vi "Live Capture Functional Stack.11.64bit.vi"() -> ()   [LabVIEW 2014]
uses:
  subvis/Stack Track.ctl
  subvis/Stack_State.ctl
  CameraControlTypeDef.ctl
  Desktop/camtiff/ctiff.llb/__CTIFFNewFileAndStyleUINT16.vi
  Desktop/camtiff/ctiff.llb/__CTIFFAddNewPageUINT16.vi
panel:
  out "Video":T1(plugin-control)
  out "Internal Line Interval":dbl
  in  "Mode":bool
  in  "Preview":bool
  in  "Capture Mode":bool
  out "Record Ready":bool
  in  "Stacks":dbl=1.0
  out "Stack Frames":i32=100
  in  "Stack Frames":i32=100
  in  "Temp":path=path "C:/temp.tmp"
  in  "Frames":i32=100
  in  "HardDisk Record":bool
  in  "Internal Line Interval":dbl
  in  "Slit Width / Lines":sgl=150.0
  in  "Camera Readout Mode":u16(ring)=12 items=["Full Frame"=1, "Slit Scanning"=12]
  in  "Readout Direction":sgl(ring)=1.0 items=["Forward"=1, "Backward"=2]
  in  "Trigger Mode":sgl(ring)=1.0 items=["Normal"=1, "Start "=6]
  in  "Trigger Source":sgl(ring)=2.0 items=["Internal"=1, "External"=2]
  out "State":T2=enum."Start Sequence"
  out "Saving":bool
  in  "AutoIncrement":bool=TRUE
  in  "Path":path=path "C:/Users/spim/Desktop/Craig Cap/temp/a.tiff"
  in  "Frames":i32=100
  out "Frame Index":i32
  out "error out":errorcluster
  in  "stop":bool
  in  "Ram Record":bool
  out "Total Frames":i32
  out "Elapsed Time":u32
  out "Software FPS":dbl
  out "Camera FPS":dbl
  in  "H Offset":i32 min=0 max=0 step=4
  in  "H Width":i32 min=4 max=2048 step=4
  out "SMD":dbl
  out "SHO":i32
  in  "V Offset":i32 min=0 max=0 step=4
  in  "V Width":i32 min=4 max=2048 step=4
  in  "Binning":u16(ring) items=["1x1"=1, "2x2"=2, "4x4"=4]
  out "SHW":i32
  out "SVO":i32
  out "SVW":i32
  in  "Scan Mode":dbl min=1.0 max=2.0 step=1.0
  in  "Exposure":dbl min=0.0010036691729323308 max=10.000004210526315 step=1e-08
  out "EXP":dbl
  out "Camera Model":string
  out "Camera Version":string
  out "Camera Serial":string
  # "Capture Mode"
  # "Preview Mode"
  # "HDD superior, will not drop frames or stacks"
  # "Change to rock switch"
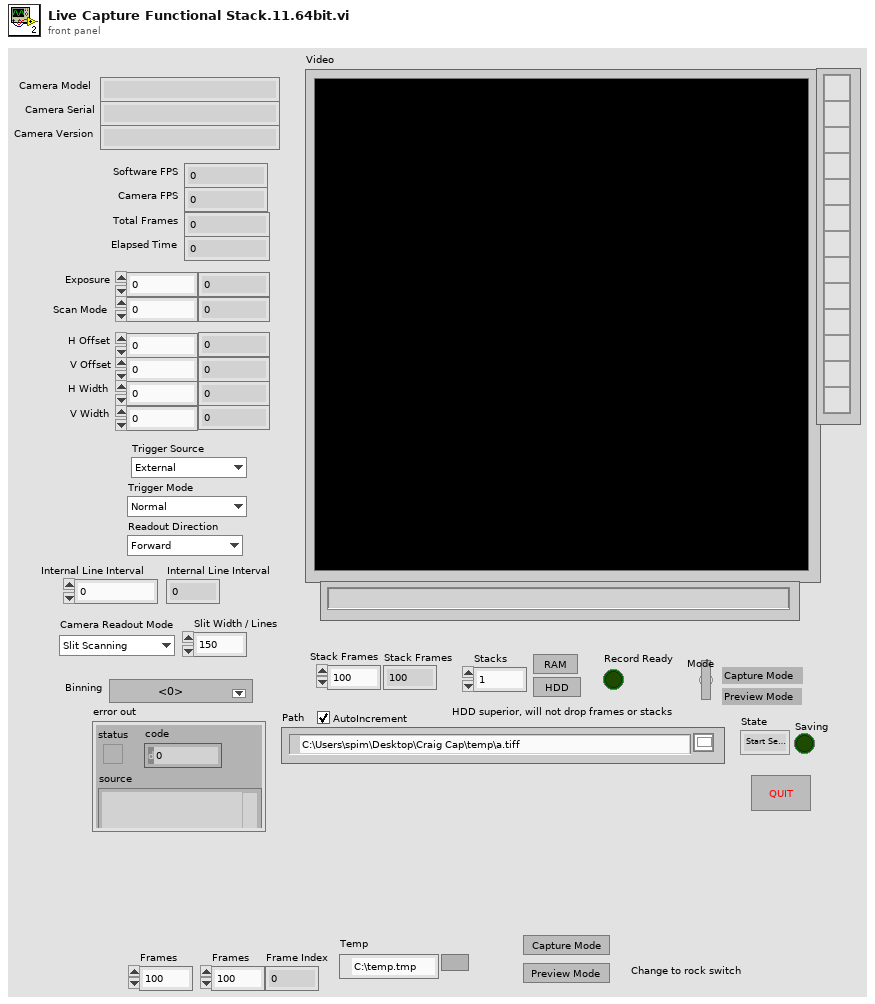
[diagram p1: front panel]
types:
  T1 = typedef "IMAQ Image.ctl" = refnum<image>
  T2 = typedef "Stack Track.ctl" = enum16{"Idle", "Start Sequence", "Read Disk", "STOP", "Collecting", "End"}
  T3 = typedef "CameraControlTypeDef.ctl" = enum16{"IntervalLineInt", "Ram Record", "HardDisk Record", "Disengage Update", "Update", "Idle", "ROI", "Binning", "Scan Mode", "Trigger Mode", "Readout Mode", "Readout Direction", "Preview"}
  T4 = typedef "Stack_State.ctl" = cluster{"State":T2, "Stack Number":i32, "Image":u16[][], "Stacks":i32}
  T5 = enum8{"Enabled", "Disabled", "Disabled and Grayed Out"}
  T6 = typedef "Image Type" = u32
  T7 = cluster{"Model":string, "Camera ID":string, "Firmware":string}
  T8 = cluster{"Value":i32, "Minimum":i32, "Maximum":i32, "Increment":i32}
  T9 = cluster{"height":u32, "width":u32, "datatype":u32}
  T10 = cluster{"H Offset":i32, "V Offset":i32, "H Width":i32, "V Width":i32}
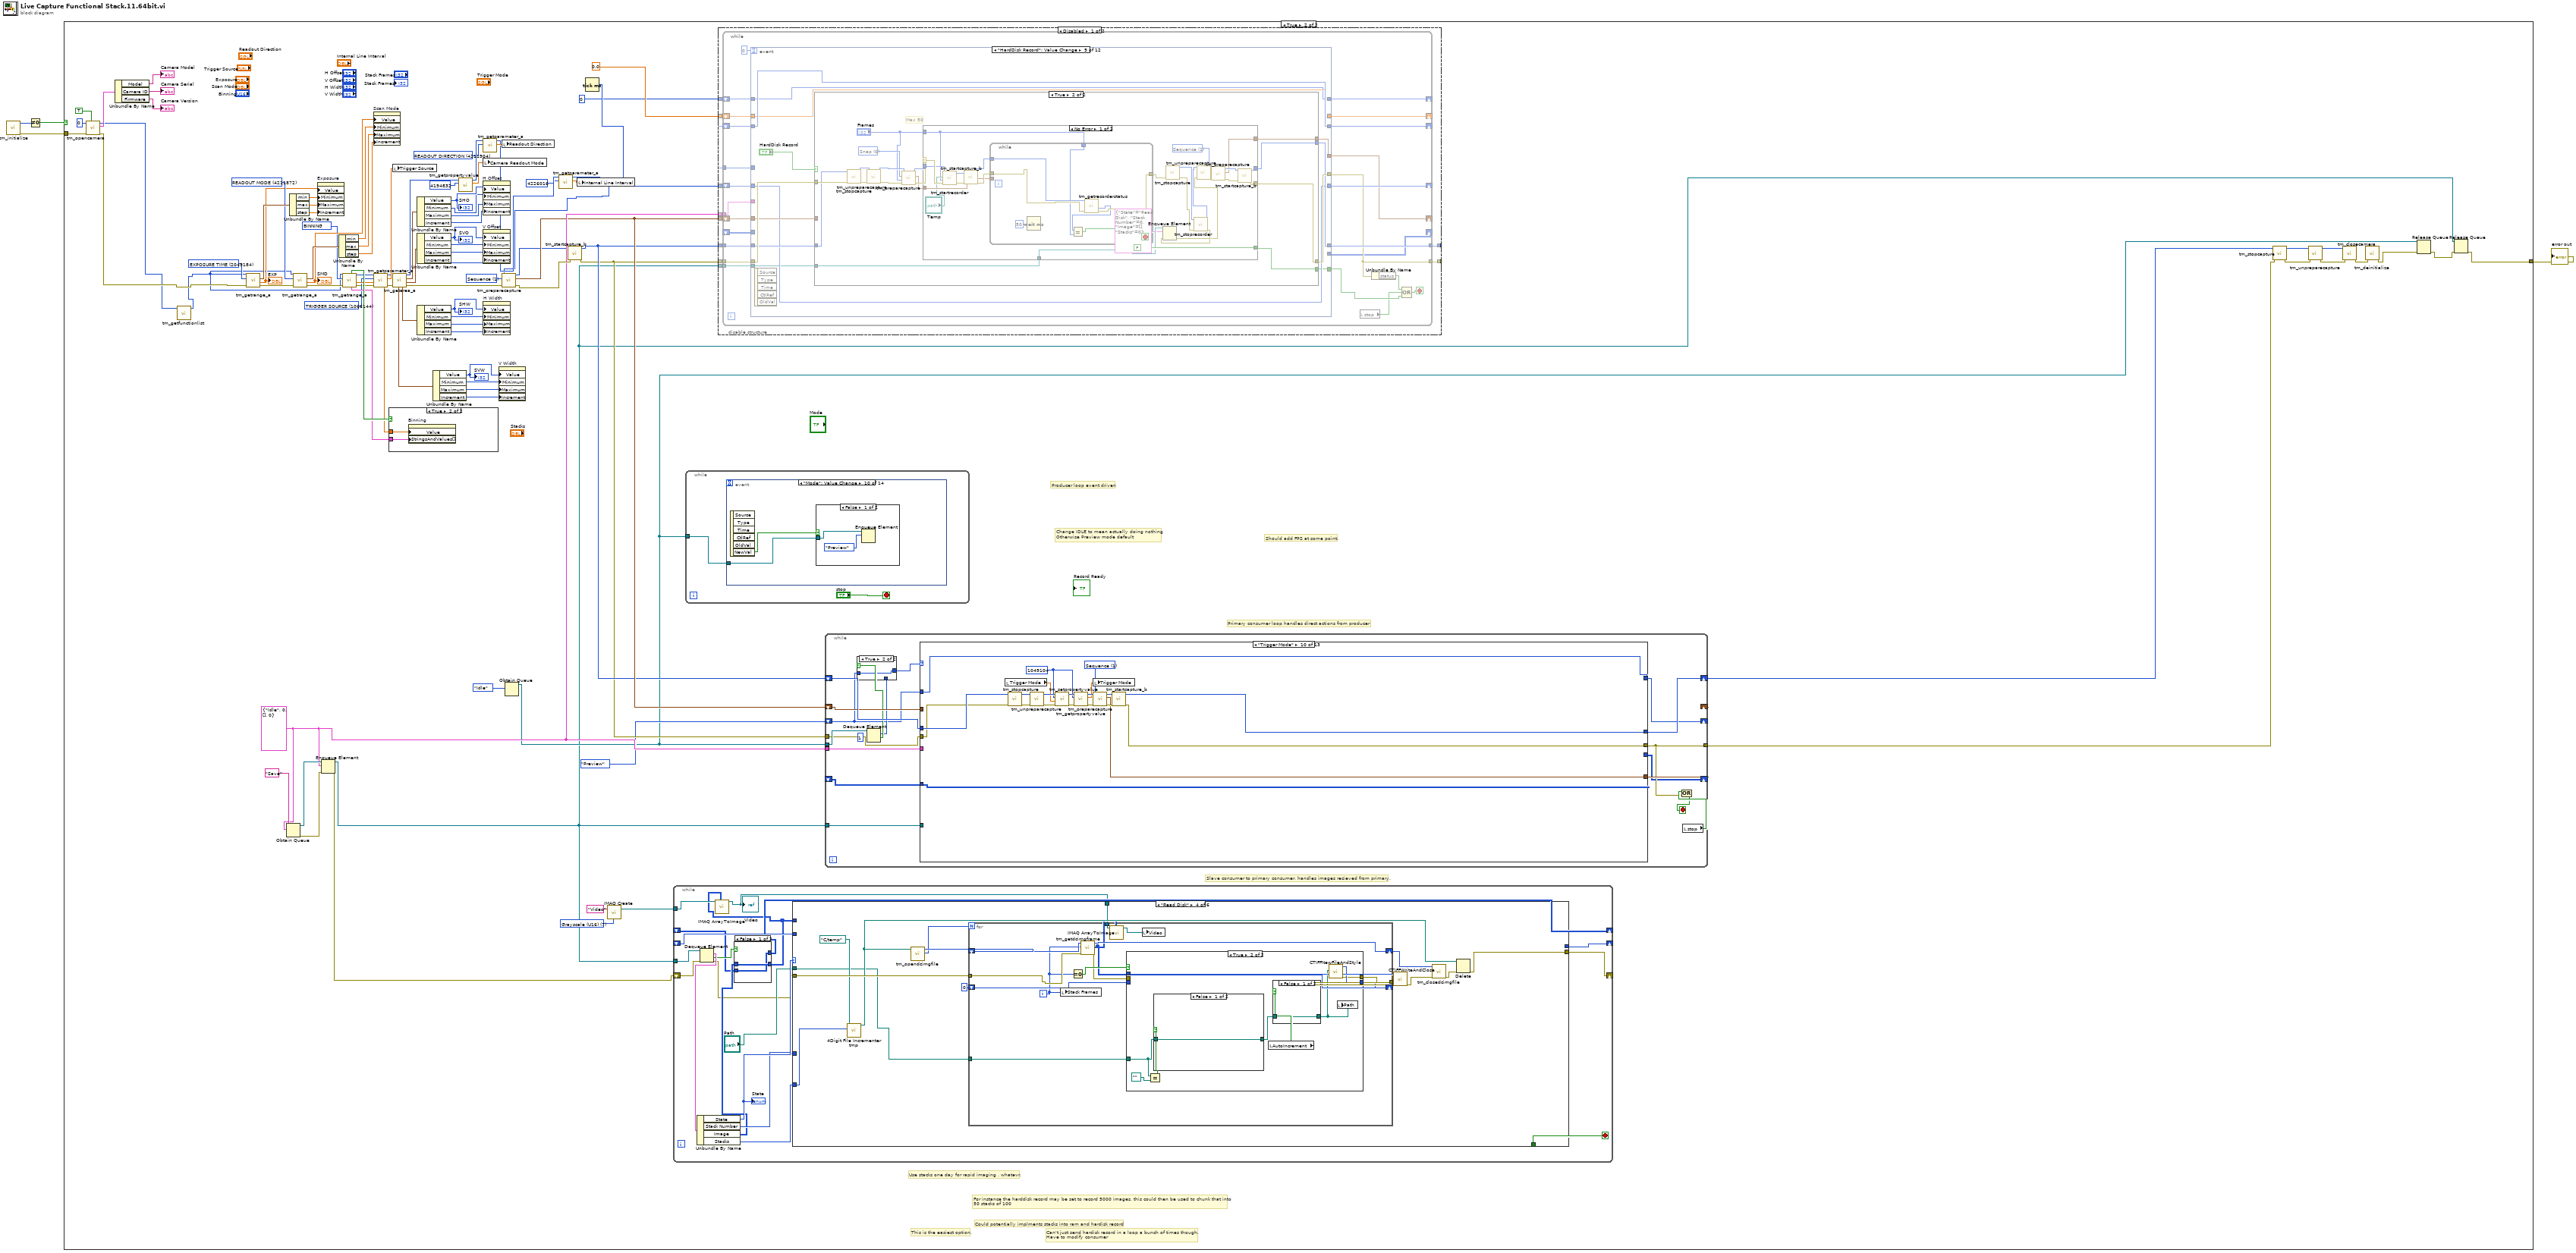
[diagram p0: block diagram]
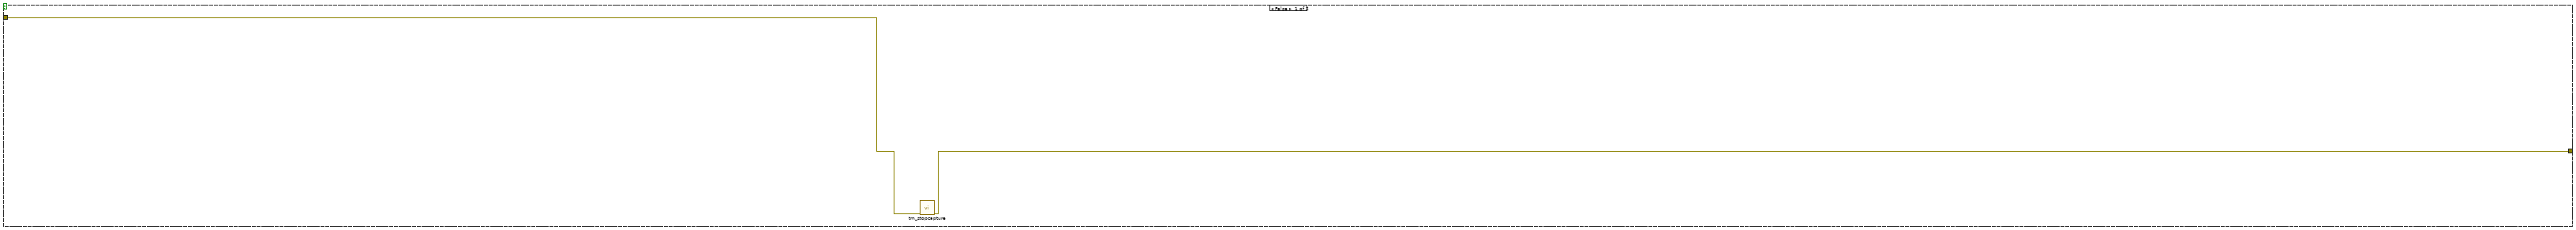
[diagram p2: hidden frame]
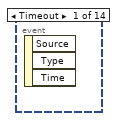
[diagram p3: hidden frame]
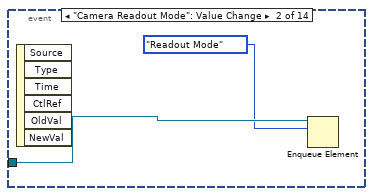
[diagram p4: hidden frame]
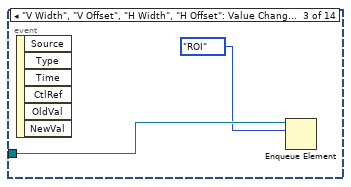
[diagram p5: hidden frame]
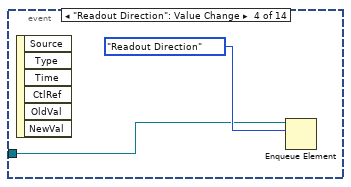
[diagram p6: hidden frame]
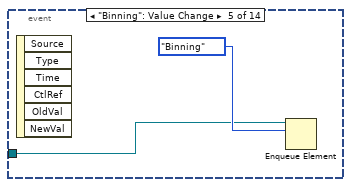
[diagram p7: hidden frame]
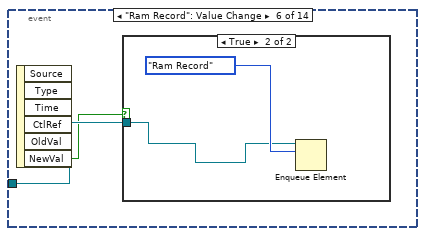
[diagram p8: hidden frame]
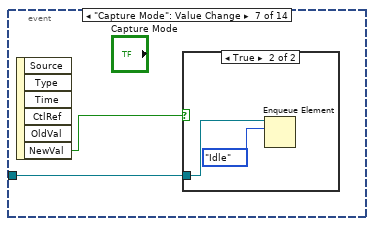
[diagram p10: hidden frame]
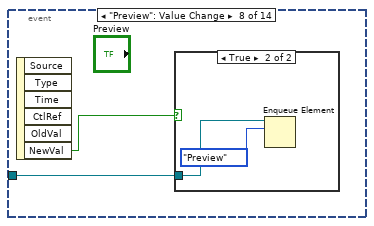
[diagram p12: hidden frame]
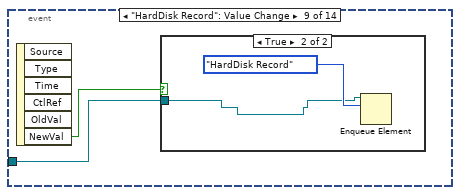
[diagram p14: hidden frame]
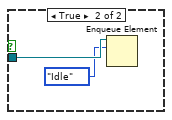
[diagram p16: hidden frame]
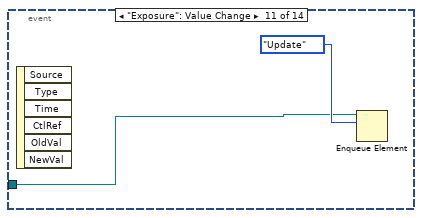
[diagram p17: hidden frame]
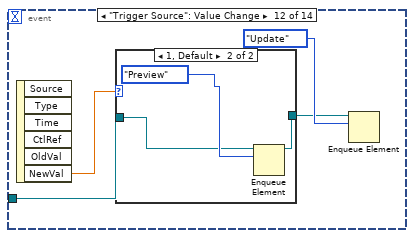
[diagram p18: hidden frame]
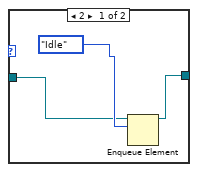
[diagram p19: hidden frame]
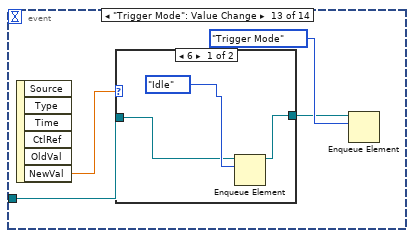
[diagram p20: hidden frame]
diagram:
  n1 = call <userlib>:"tm_initialize.vi"() -> ("error out"=w2:errorcluster, "Number Of Cameras"=w1:u32)  [unwired: 8 in, 2 out]
  n2 = Not Equal To 0?(x=w1) -> (x != 0?=w4:bool)
  n3 = case shown="True" w4 {
    tunnel: [w5 w19] -> w3
    tunnel: w2 -> [w6 w102]
    frame False {
      n4 = call <userlib>:"tm_stopcapture.vi"("error in (no error)"=w6) -> ("error out"=w5:errorcluster)  [unwired: 9 in, 1 out]
    }
    frame True {
      w9 = T6 7 items=["Grayscale (U8)", "Grayscale (I16)", "Grayscale (SGL)", "Complex (CSG)", "RGB (U32)", "HSL (U32)", "RGB (U64)", "Grayscale (U16)"] ("Image Type")
      w37 = u32 4211904 items=["SENSOR MODE"=4212128, "CCD MODE"=4212384, "READOUT MODE"=4211872, "ACTIVE VIEW INDEX"=4343136, "BITS PER CHANNEL"=4342976, "IMAGE PIXEL TYPE"=4343296, "BINNING"=4215968, "EXPOSURE TIME"=2049184, "CONTRAST GAIN"=3163312, "CONTRAST OFFSET"=3163328, "LIGHT MODE"=2114720, "SENSITIVITY"=2114992, "PHOTON IMAGING MODE"=2115200, "HIGH DYNAMIC RANGE MODE"=3163360, "WHITE BALANCE"=3163568, "TEMPERATURE"=2115232, "TEMPERATURE TARGET"=2115264, "SENSOR COOLER FAN"=2115296, "LINEBUNDLE HEIGHT"=4212192, "MECHANICAL SHUTTER"=2115488, "BACK FOCUS POSITION"=8422304, "TRIGGER CONNECTOR"=1066432, "TRIGGER SOURCE"=1066144, "OUTPUT TRIGGER SOURCE"=1852576, "TRIGGER GLOBAL EXPOSURE"=2049680, "FIRST TRIGGER BEHAVIOR"=2049696, "CHANNEL SYNC"=1852352, "READOUT DIRECTION"=4211904, "PRE HSYNC COUNT"=1852704] ("Parameter")
      w46 = u32 1066144 items=["SENSOR MODE"=4212128, "CCD MODE"=4212384, "READOUT MODE"=4211872, "ACTIVE VIEW INDEX"=4343136, "BITS PER CHANNEL"=4342976, "IMAGE PIXEL TYPE"=4343296, "BINNING"=4215968, "EXPOSURE TIME"=2049184, "CONTRAST GAIN"=3163312, "CONTRAST OFFSET"=3163328, "LIGHT MODE"=2114720, "SENSITIVITY"=2114992, "PHOTON IMAGING MODE"=2115200, "HIGH DYNAMIC RANGE MODE"=3163360, "WHITE BALANCE"=3163568, "TEMPERATURE"=2115232, "TEMPERATURE TARGET"=2115264, "SENSOR COOLER FAN"=2115296, "LINEBUNDLE HEIGHT"=4212192, "MECHANICAL SHUTTER"=2115488, "BACK FOCUS POSITION"=8422304, "TRIGGER CONNECTOR"=1066432, "TRIGGER SOURCE"=1066144, "OUTPUT TRIGGER SOURCE"=1852576, "TRIGGER GLOBAL EXPOSURE"=2049680, "FIRST TRIGGER BEHAVIOR"=2049696, "CHANNEL SYNC"=1852352, "READOUT DIRECTION"=4211904, "PRE HSYNC COUNT"=1852704] ("Parameter")
      w32 = T4 {"State"=enum."Idle", "Stack Number"=0, "Image"=[], "Stacks"=0} ("input cluster")
      w51 = u32 2049184 items=["BINNING"=4215968, "BITS PER CHANNEL"=4342976, "ACTIVE VIEW INDEX"=4343136, "CCD MODE"=4212384, "SENSOR MODE"=4212128, "READOUT MODE"=4211872, "EXPOSURE TIME"=2049184, "CONTRAST GAIN"=3163312, "CONTRAST OFFSET"=3163328, "LIGHT MODE"=2114720, "SENSITIVITY"=2114992, "WHITE BALANCE"=3163568, "PHOTON IMAGING MODE"=2115200, "HIGH DYNAMIC RANGE MODE"=3163360, "TRIGGER SOURCE"=1066144, "TRIGGER ACTIVE"=1066160, "TRIGGER MODE"=1066400, "TRIGGER POLARITY"=1066416, "TRIGGER GLOBAL EXPOSURE"=2049680, "FIRST TRIGGER BEHAVIOR"=2049696, "TRIGGER TIMES"=1066448, "OUTPUT TRIGGER POLARITY"=1852592, "OUTPUT TRIGGER DELAY"=1852624, "OUTPUT TRIGGER PERIOD"=1852640, "TEMPERATURE"=2115232, "TEMPERATURE TARGET"=2115264, "SENSOR COOLER FAN"=2115296, "MECHANICAL SHUTTER"=2115488, "BACK FOCUS POSITION"=8422304, "FRAMEBUNDLE MODE"=4346784, "FRAMEBUNDLE NUMBER"=4346800, "LINEBUNDLE HEIGHT"=4212192, "TRIGGER CONNECTOR"=1066432, "IMAGE PIXEL TYPE"=4343296, "OUTPUT TRIGGER KIND"=1852656, "READOUT DIRECTION"=4211904, "CHANNEL SYNC"=1852352] ("Parameter")
      w52 = u32 4211872 items=["BINNING"=4215968, "BITS PER CHANNEL"=4342976, "ACTIVE VIEW INDEX"=4343136, "CCD MODE"=4212384, "SENSOR MODE"=4212128, "READOUT MODE"=4211872, "EXPOSURE TIME"=2049184, "CONTRAST GAIN"=3163312, "CONTRAST OFFSET"=3163328, "LIGHT MODE"=2114720, "SENSITIVITY"=2114992, "WHITE BALANCE"=3163568, "PHOTON IMAGING MODE"=2115200, "HIGH DYNAMIC RANGE MODE"=3163360, "TRIGGER SOURCE"=1066144, "TRIGGER ACTIVE"=1066160, "TRIGGER MODE"=1066400, "TRIGGER POLARITY"=1066416, "TRIGGER GLOBAL EXPOSURE"=2049680, "FIRST TRIGGER BEHAVIOR"=2049696, "TRIGGER TIMES"=1066448, "OUTPUT TRIGGER POLARITY"=1852592, "OUTPUT TRIGGER DELAY"=1852624, "OUTPUT TRIGGER PERIOD"=1852640, "TEMPERATURE"=2115232, "TEMPERATURE TARGET"=2115264, "SENSOR COOLER FAN"=2115296, "MECHANICAL SHUTTER"=2115488, "BACK FOCUS POSITION"=8422304, "FRAMEBUNDLE MODE"=4346784, "FRAMEBUNDLE NUMBER"=4346800, "LINEBUNDLE HEIGHT"=4212192, "TRIGGER CONNECTOR"=1066432, "IMAGE PIXEL TYPE"=4343296, "OUTPUT TRIGGER KIND"=1852656, "READOUT DIRECTION"=4211904, "CHANNEL SYNC"=1852352] ("Parameter")
      w53 = u32 4215968 items=["BINNING"=4215968, "BITS PER CHANNEL"=4342976, "ACTIVE VIEW INDEX"=4343136, "CCD MODE"=4212384, "SENSOR MODE"=4212128, "READOUT MODE"=4211872, "EXPOSURE TIME"=2049184, "CONTRAST GAIN"=3163312, "CONTRAST OFFSET"=3163328, "LIGHT MODE"=2114720, "SENSITIVITY"=2114992, "WHITE BALANCE"=3163568, "PHOTON IMAGING MODE"=2115200, "HIGH DYNAMIC RANGE MODE"=3163360, "TRIGGER SOURCE"=1066144, "TRIGGER ACTIVE"=1066160, "TRIGGER MODE"=1066400, "TRIGGER POLARITY"=1066416, "TRIGGER GLOBAL EXPOSURE"=2049680, "FIRST TRIGGER BEHAVIOR"=2049696, "TRIGGER TIMES"=1066448, "OUTPUT TRIGGER POLARITY"=1852592, "OUTPUT TRIGGER DELAY"=1852624, "OUTPUT TRIGGER PERIOD"=1852640, "TEMPERATURE"=2115232, "TEMPERATURE TARGET"=2115264, "SENSOR COOLER FAN"=2115296, "MECHANICAL SHUTTER"=2115488, "BACK FOCUS POSITION"=8422304, "FRAMEBUNDLE MODE"=4346784, "FRAMEBUNDLE NUMBER"=4346800, "LINEBUNDLE HEIGHT"=4212192, "TRIGGER CONNECTOR"=1066432, "IMAGE PIXEL TYPE"=4343296, "OUTPUT TRIGGER KIND"=1852656, "READOUT DIRECTION"=4211904, "CHANNEL SYNC"=1852352] ("Parameter")
      w98 = 1 items=["Snap", "Sequence"] ("Capture mode")
      # "Can't just send hardisk record in a loop a bunch of times though.\nHave to modify consumer"
      # "This is the easiest option."
      # "Could potentially implments stacks into ram and hardisk record"
      # "For instance the harddisk record may be set to record 5000 images, this could then be used to chunk that into\n50 stacks of 100"
      # "Use stacks one day for rapid imaging , whatevr."
      # "Change IDLE to mean actually doing nothing\nOtherwise Preview mode default"
      # "Slave consumer to primary consumer, handles images recieved from primary."
      # "Primary consumer loop handles direct actions from producer"
      # "Producer loop event driven"
      # "Should add FPS at some point."
      n5 = call <userlib>:"tm_opencamera.vi"("Force Open"=TRUE, "error in (no error)"=w102, "Camera Index"=u32 0) -> ("error out"=w33:errorcluster, "Camera Details"=w65:T7, "Handle out"=w17:u32)  [unwired: 6 in]
      n6 = Unbundle By Name(w65) -> ("Model"=→"Camera Model":string, "Camera ID"=→"Camera Serial":string, "Firmware"=→"Camera Version":string)
      n7 = call <userlib>:"tm_getfunctionlist.vi"("Handle in"=w17) -> ("Handle out"=w16:u32)  [unwired: 8 in, 2 out]
      n8 = call <userlib>:"tm_getrange_a.vi"("error in (no error)"=w33, "Parameter"=w51, "Handle in"=w16) -> ("error out"=w60:errorcluster, "default"=w49:dbl, "Range"=w61:cluster{"min":dbl, "max":dbl, "step":dbl})  [unwired: 2 in, 4 out]
      "EXP" <- w49
      n9 = Obtain Queue(name (unnamed)="Save", element data type=w32) -> (queue out=w35:refnum<queue>, error out=w14:errorcluster)  [unwired: 3 in, 1 out]
      n10 = Unbundle By Name(w61) -> ("min"=w96:dbl, "max"=w95:dbl, "step"=w94:dbl)
      n11 = call <userlib>:"tm_getrange_a.vi"("error in (no error)"=w60, "Parameter"=w52, "Handle in"=w16) -> ("error out"=w57:errorcluster, "default"=w58:dbl, "Range"=w59:cluster{"min":dbl, "max":dbl, "step":dbl})  [unwired: 2 in, 4 out]
      "SMD" <- w58
      n12 = property on="Exposure" class="DigNum (strict)"("Value"=w49, "Minimum"=w96, "Maximum"=w95, "Increment"=w94) -> ()  [unwired: 2 in, 2 out]
      n13 = Enqueue Element(queue=w35, element=w32, error in (no error)=w14) -> (queue out=w18:refnum<queue>, error out=w13:errorcluster)  [unwired: 1 in, 1 out]
      n14 = Unbundle By Name(w59) -> ("min"=w93:dbl, "max"=w92:dbl, "step"=w91:dbl)
      n15 = call <userlib>:"tm_getrange_a.vi"("error in (no error)"=w57, "Parameter"=w53, "Handle in"=w16) -> ("error out"=w43:errorcluster, "default"=w55:dbl, "Handle out"=w45:u32, "Value Names"=w54:cluster{"Name":string, "Value":dbl}[], "Writable"=w56:bool)  [unwired: 2 in, 2 out]
      n16 = property on="Scan Mode" class="DigNum (strict)"("Value"=w58, "Minimum"=w93, "Maximum"=w92, "Increment"=w91) -> ()  [unwired: 2 in, 2 out]
      n17 = call <userlib>:"tm_getparameter_a.vi"("error in (no error)"=w43, "Parameter"=w46, "Handle in"=w45) -> ("error out"=w42:errorcluster, "Value out"=w47:dbl, "Handle out"=w44:u32)  [unwired: 6 in]
      n18 = case shown="True" w56 {
        tunnel: w54 -> [_ w1206]
        tunnel: w55 -> [_ w1205]
        frame False {
        }
        frame True {
          n19 = property on="Binning" class="Ring (strict)"("Value"=w1205, "StringsAndValues[]"=w1206) -> ()  [unwired: 2 in, 2 out]
        }
      }
      n20 = local write "Trigger Source"(w47) -> ()
      n21 = call <userlib>:"tm_getarea_a.vi"("error in (no error)"=w42, "Handle in"=w44) -> ("error out"=w48:errorcluster, "V Offset"=w90:T8, "H Offset"=w71:T8, "Handle out"=w39:u32, "H Width"=w89:T8, "V Width"=w88:T8)  [unwired: 4 in]
      n22 = Unbundle By Name(w71) -> ("Value"=w70:i32, "Minimum"=w69:i32, "Maximum"=w68:i32, "Increment"=w67:i32)
      "SHO" <- w70
      n23 = Unbundle By Name(w90) -> ("Value"=w78:i32, "Minimum"=w87:i32, "Maximum"=w86:i32, "Increment"=w85:i32)
      "SVO" <- w78
      n24 = Unbundle By Name(w89) -> ("Value"=w77:i32, "Minimum"=w84:i32, "Maximum"=w83:i32, "Increment"=w82:i32)
      "SHW" <- w77
      n25 = Unbundle By Name(w88) -> ("Value"=w76:i32, "Minimum"=w81:i32, "Maximum"=w80:i32, "Increment"=w79:i32)
      "SVW" <- w76
      n26 = call <userlib>:"tm_getpropertyvalue.vi"("Property ID"=u32 4194832, "Handle in"=w39) -> ("Value in"=w40:sgl, "Handle out"=w38:u32)  [unwired: 7 in, 1 out]
      n27 = call <userlib>:"tm_getparameter_a.vi"("Parameter"=w37, "Handle in"=w38) -> ("Value out"=w36:dbl, "Handle out"=w23:u32)  [unwired: 7 in, 1 out]
      n28 = local write "Camera Readout Mode"(w40) -> ()
      n29 = property on="H Offset" class="DigNum (strict)"("Value"=w70, "Minimum"=w69, "Maximum"=w68, "Increment"=w67) -> ()  [unwired: 2 in, 2 out]
      n30 = property on="V Offset" class="DigNum (strict)"("Value"=w78, "Minimum"=w87, "Maximum"=w86, "Increment"=w85) -> ()  [unwired: 2 in, 2 out]
      n31 = property on="H Width" class="DigNum (strict)"("Value"=w77, "Minimum"=w84, "Maximum"=w83, "Increment"=w82) -> ()  [unwired: 2 in, 2 out]
      n32 = property on="V Width" class="DigNum (strict)"("Value"=w76, "Minimum"=w81, "Maximum"=w80, "Increment"=w79) -> ()  [unwired: 2 in, 2 out]
      n33 = local write "Readout Direction"(w36) -> ()
      n34 = Obtain Queue(element data type=CameraControlTypeDef."Idle" ("Enum")) -> (queue out=w21:refnum<queue>)  [unwired: 4 in, 2 out]
      n35 = call <userlib>:"tm_getparameter_a.vi"("Parameter"=4226016, "Handle in"=w23) -> ("Value out"=w11:dbl, "Handle out"=w12:u32)  [unwired: 7 in, 1 out]
      n36 = call <userlib>:"tm_preparecapture.vi"("error in (no error)"=w48, "Capture mode"=w98, "Handle in"=w12) -> ("error out"=w34:errorcluster, "Buffer Info"=w31:T9, "Handle out"=w24:u32)  [unwired: 5 in, 1 out]
      n37 = call <userlib>:"tm_startcapture_b.vi"("error in (no error)"=w34, "Handle in"=w24) -> ("error out"=w29:errorcluster, "Handle out"=w30:u32)  [unwired: 8 in]
      n38 = local write "Internal Line Interval"(w11) -> ()
      n39 = Tick Count (ms)() -> (millisecond timer value=w97:u32)
      n40 = call "IMAQ Create"("Image Name"="Video", "Image Type"=w9) -> ("New Image"=w8:T1)  [unwired: 3 in, 1 out]
      n41 = while {
        tunnel: w18 -> [w1119]
        shift-right: [w1115] -> _
        shift-left: _ -> [w1113]
        shift-right: [w1112] -> _
        shift-left: w13 -> [w1106]
        shift-right: [w1110] -> _
        shift-left: _ -> [w1107]
        tunnel: w8 -> [w1103]
        stop <- w1114 stop-if-true
        n42 = Dequeue Element(queue=w1119, error in (no error)=w1106) -> (element=w1118:T4, timed out?=w1108:bool, error out=w1105:errorcluster)  [unwired: 1 in, 1 out]
        n43 = Unbundle By Name(w1118) -> ("State"=w1117:T2, "Stack Number"=w1116:i32, "Image"=w1109:u16[][], "Stacks"=w1104:i32)
        "State" <- w1117
        n44 = case shown="False" w1108 {
          tunnel: w1109 -> [w1121 w1123]
          tunnel: [w1121 w1122] -> w1102
          tunnel: [w1120 w1123] -> w1110
          tunnel: w1107 -> [w1120 w1122]
          frame False {
          }
          frame True {
          }
        }
        n45 = call "IMAQ ArrayToImage"("Image Pixels (U16)"=w1102, "Image"=w1103) -> ("Image Out"=w1101:T1)  [unwired: 8 in, 1 out]
        "Video" <- w1101
        n46 = case shown="\"Read Disk\"" w1117 {
          tunnel: w1116 -> [_ _ _ _ _ _]
          tunnel: [w1126 w1143 _ _ _ _] -> w1115
          tunnel: w1113 -> [_ w1144 w1150 _ _ _]
          tunnel: [FALSE _ _ _ TRUE _] -> w1114
          tunnel: w1102 -> [w1124 w1145 _ _ _ _]
          tunnel: w1105 -> [_ w1142 w1148 w1164 w1202 w1204]
          tunnel: [w1127 w1141 w1149 w1161 w1202 w1204] -> w1112
          tunnel: "Path" -> [w1130 _ _ w1154 _ _]
          tunnel: w1104 -> [_ _ _ w1157 _ _]
          tunnel: w1101 -> [_ _ _ w1153 _ _]
          frame "Start Sequence" {
            # "Public tiff library"
            # "Get path and open file"
            n47 = Equal?(x=w1130, y=path "") -> (x = y?=w1132:bool)
            n48 = case shown="True" w1132 {
              tunnel: w1130 -> [w1134 _]
              tunnel: [w1134 w1137] -> w1129
              frame False {
              }
              frame True {
                n49 = call "File Dialog"("pattern (all files)"=".tiff", "pattern label"="Tiff Image") -> ("selected path"=w1137:path)  [unwired: 10 in, 3 out]
              }
            }
            n50 = case shown="True" "AutoIncrement" {
              tunnel: w1129 -> [w1138 w1140]
              tunnel: [w1138 w1139] -> w1125
              frame False {
              }
              frame True {
                n51 = call "4Digit File Incrementer.vi"("path"=w1140) -> ("appended path"=w1139:path)  [unwired: 10 in]
              }
            }
            n52 = local write "Path"(w1125) -> ()
            n53 = call-poly "CTIFFNewFileAndStyle.vi"("image"=w1124, "output_file"=w1125) -> ("error"=w1127:errorcluster, "CTIFF"=w1126:i64)  [unwired: 8 in]
          }
          frame "Collecting" {
            # "Add Image to write scan line"
            n54 = call-poly "CTIFFAddNewPage.vi"("error"=w1142, "image"=w1145, "CTIFF"=w1144) -> ("error"=w1141:errorcluster, "CTIFF"=w1143:i64)  [unwired: 7 in]
            n55 = property on="Ram Record" class="Bool (strict)"("DisabledEnum"=T5."Disabled and Grayed Out" ("Disabled"), "BoolText.Text"="Saving" ("Boolean Text.Text")) -> ()  [unwired: 2 in, 2 out]
          }
          frame "End" {
            (unwired) FALSE
            # "Close image file, reset capturing button"
            n56 = call "CTIFFWriteAndClose.vi"("error"=w1148, "CTIFF"=w1150) -> ("error"=w1149:errorcluster)  [unwired: 9 in]
            n57 = property on="Ram Record" class="Bool (strict)"("BoolText.Text"="RAM" ("Boolean Text.Text"), "DisabledEnum"=T5."Enabled" ("Disabled")) -> ()  [unwired: 2 in, 2 out]
          }
          frame "Read Disk" {
            n58 = call "4Digit File Incrementer tmp.vi"("Number"=w1157, "path"=path "C:/temp" ("Temp 2")) -> ("appended path"=w1155:path)  [unwired: 9 in]
            n59 = call <userlib>:"tm_opendcimgfile.vi"("Path"=w1155) -> ("Total Frames"=w1166:i32, "File Handle"=w1167:u32)  [unwired: 8 in, 1 out]
            n60 = for {
              N: w1166 -> [_]
              shift-right: [w1176] -> w1162
              shift-left: i64 0 ("CTIFF") -> [w1177]
              tunnel: [w1175] -> w1163
              tunnel: w1164 -> [w1174]
              shift-right: [w1179] -> w1158
              shift-left: w1167 -> [w1180]
              tunnel: w1154 -> [w1171]
              tunnel: w1153 -> [w1169]
              i -> [w1172]
              n61 = local write "Stack Frames"(w1172) -> ()
              n62 = Equal To 0?(x=w1172) -> (x = 0?=w1178:bool)
              n63 = call <userlib>:"tm_getdcimgframe.vi"("error in (no error)"=w1174, "Frame Index"=w1172, "File Handle in"=w1180) -> ("error out"=w1173:errorcluster, "Data"=w1168:u16[][], "File Handle out"=w1179:u32)  [unwired: 5 in, 1 out]
              n64 = call "IMAQ ArrayToImage"("Image Pixels (U16)"=w1168, "Image"=w1169) -> ("Image Out"=w1170:T1)  [unwired: 8 in, 1 out]
              n65 = case shown="True" w1178 {
                tunnel: w1168 -> [w1181 w1194]
                tunnel: w1177 -> [w1185 _]
                tunnel: [w1184 w1193] -> w1176
                tunnel: [w1183 w1192] -> w1175
                tunnel: w1173 -> [w1182 _]
                tunnel: w1171 -> [_ w1187]
                frame False {
                  n66 = call-poly "CTIFFAddNewPage.vi"("error"=w1182, "image"=w1181, "CTIFF"=w1185) -> ("error"=w1183:errorcluster, "CTIFF"=w1184:i64)  [unwired: 7 in]
                }
                frame True {
                  n67 = Equal?(x=w1187, y=path "") -> (x = y?=w1188:bool)
                  n68 = case shown="False" w1188 {
                    tunnel: [w1195 w1196] -> w1191
                    tunnel: w1187 -> [w1195 _]
                    frame False {
                    }
                    frame True {
                      n69 = call "File Dialog2"("pattern (all files)"=".tiff", "pattern label"="Tiff Image") -> ("selected path"=w1196:path)  [unwired: 10 in, 3 out]
                    }
                  }
                  n70 = local read "AutoIncrement"() -> (w1190:bool)
                  n71 = case shown="False" w1190 {
                    tunnel: w1191 -> [w1199 w1200]
                    tunnel: [w1199 w1201] -> w1186
                    frame False {
                    }
                    frame True {
                      n72 = call "4Digit File Incrementer.vi"("path"=w1200) -> ("appended path"=w1201:path)  [unwired: 10 in]
                    }
                  }
                  n73 = call-poly "CTIFFNewFileAndStyle.vi"("image"=w1194, "output_file"=w1186) -> ("error"=w1192:errorcluster, "CTIFF"=w1193:i64)  [unwired: 8 in]
                  n74 = local write "Path"(w1186) -> ()
                }
              }
              n75 = local write "Video"(w1170) -> ()
            }
            n76 = call "CTIFFWriteAndClose.vi"("error"=w1163, "CTIFF"=w1162) -> ("error"=w1160:errorcluster)  [unwired: 9 in]
            n77 = call <userlib>:"tm_closedcimgfile.vi"("error in (no error)"=w1160, "File Handle"=w1158) -> ("error out"=w1159:errorcluster)  [unwired: 9 in]
            n78 = Delete(path (use dialog)=w1155, error in=w1159) -> (error out=w1161:errorcluster)  [unwired: 3 in, 2 out]
          }
          frame "STOP" {
          }
          frame "Idle" {
          }
        }
      }
      n79 = while {
        tunnel: w21 -> [w104]
        stop <- "stop" stop-if-true
        n80 = event shown="[9] \"Mode\": Value Change" {
          selector: _ -> [_ _ _ _ _ _ _ _ _ _ _ _ _ _]
          dyn-events: _ -> [_ _ _ _ _ _ _ _ _ _ _ _ _ _]
          timeout: _ -> [_ _ _ _ _ _ _ _ _ _ _ _ _ _]
          tunnel: w104 -> [_ w106 w108 w109 w111 w114 w117 w121 w126 w129 w135 w139 w149 w159]
          event Timeout {
            n81 = event-data() -> ()  [unwired: 1 in, 3 out]
          }
          event "Camera Readout Mode": Value Change {
            n82 = event-data() -> ()  [unwired: 1 in, 6 out]
            n83 = Enqueue Element(queue=w106, element=CameraControlTypeDef."Readout Mode" ("Enum")) -> ()  [unwired: 2 in, 3 out]
          }
          event "V Width", "V Offset", "H Width", "H Offset": Value Change {
            n84 = event-data() -> ()  [unwired: 1 in, 6 out]
            n85 = Enqueue Element(queue=w108, element=CameraControlTypeDef."ROI" ("Enum")) -> ()  [unwired: 2 in, 3 out]
          }
          event "Readout Direction": Value Change {
            n86 = event-data() -> ()  [unwired: 1 in, 6 out]
            n87 = Enqueue Element(queue=w109, element=CameraControlTypeDef."Readout Direction" ("Enum")) -> ()  [unwired: 2 in, 3 out]
          }
          event "Binning": Value Change {
            n88 = event-data() -> ()  [unwired: 1 in, 6 out]
            n89 = Enqueue Element(queue=w111, element=CameraControlTypeDef."Binning" ("Enum")) -> ()  [unwired: 2 in, 3 out]
          }
          event "Ram Record": Value Change {
            n90 = event-data() -> ("NewVal"=w113:bool)  [unwired: 1 in, 5 out]
            n91 = case shown="True" w113 {
              tunnel: w114 -> [_ w115]
              frame False {
              }
              frame True {
                n92 = Enqueue Element(queue=w115, element=CameraControlTypeDef."Ram Record" ("Enum")) -> ()  [unwired: 2 in, 3 out]
              }
            }
          }
          event "Capture Mode": Value Change {
            n93 = event-data() -> ("NewVal"=w118:bool)  [unwired: 1 in, 5 out]
            n94 = case shown="True" w118 {
              tunnel: w117 -> [_ w120]
              frame False {
              }
              frame True {
                n95 = Enqueue Element(queue=w120, element=CameraControlTypeDef."Idle") -> ()  [unwired: 2 in, 3 out]
              }
            }
          }
          event "Preview": Value Change {
            n96 = event-data() -> ("NewVal"=w122:bool)  [unwired: 1 in, 5 out]
            n97 = case shown="True" w122 {
              tunnel: w121 -> [_ w124]
              frame False {
              }
              frame True {
                n98 = Enqueue Element(queue=w124, element=CameraControlTypeDef."Preview") -> ()  [unwired: 2 in, 3 out]
              }
            }
          }
          event "HardDisk Record": Value Change {
            n99 = event-data() -> ("NewVal"=w125:bool)  [unwired: 1 in, 5 out]
            n100 = case shown="True" w125 {
              tunnel: w126 -> [_ w127]
              frame False {
              }
              frame True {
                n101 = Enqueue Element(queue=w127, element=CameraControlTypeDef."HardDisk Record" ("Enum")) -> ()  [unwired: 2 in, 3 out]
              }
            }
          }
          event "Mode": Value Change {
            n102 = event-data() -> ("NewVal"=w130:bool)  [unwired: 1 in, 5 out]
            n103 = case shown="False" w130 {
              tunnel: w129 -> [w131 w134]
              frame False {
                n104 = Enqueue Element(queue=w131, element=CameraControlTypeDef."Preview") -> ()  [unwired: 2 in, 3 out]
              }
              frame True {
                n105 = Enqueue Element(queue=w134, element=CameraControlTypeDef."Idle") -> ()  [unwired: 2 in, 3 out]
              }
            }
          }
          event "Exposure": Value Change {
            n106 = event-data() -> ()  [unwired: 1 in, 6 out]
            n107 = Enqueue Element(queue=w135, element=CameraControlTypeDef."Update" ("Enum")) -> ()  [unwired: 2 in, 3 out]
          }
          event "Trigger Source": Value Change {
            n108 = event-data() -> ("NewVal"=w137:sgl)  [unwired: 1 in, 5 out]
            n109 = case shown="1, Default" w137 {
              tunnel: w139 -> [w142 w145]
              tunnel: [w141 w144] -> w138
              frame 2 {
                n110 = Enqueue Element(queue=w142, element=CameraControlTypeDef."Idle" ("Enum")) -> (queue out=w141:refnum<queue>)  [unwired: 2 in, 2 out]
              }
              frame 1, Default {
                n111 = Enqueue Element(queue=w145, element=CameraControlTypeDef."Preview" ("Enum")) -> (queue out=w144:refnum<queue>)  [unwired: 2 in, 2 out]
              }
            }
            n112 = Enqueue Element(queue=w138, element=CameraControlTypeDef."Update" ("Enum")) -> ()  [unwired: 2 in, 3 out]
          }
          event "Trigger Mode": Value Change {
            n113 = event-data() -> ("NewVal"=w147:sgl)  [unwired: 1 in, 5 out]
            n114 = case shown="6" w147 {
              tunnel: w149 -> [w152 w155]
              tunnel: [w151 w154] -> w148
              frame 6 {
                n115 = Enqueue Element(queue=w152, element=CameraControlTypeDef."Idle" ("Enum")) -> (queue out=w151:refnum<queue>)  [unwired: 2 in, 2 out]
              }
              frame 1, Default {
                n116 = Enqueue Element(queue=w155, element=CameraControlTypeDef."Preview" ("Enum")) -> (queue out=w154:refnum<queue>)  [unwired: 2 in, 2 out]
              }
            }
            n117 = Enqueue Element(queue=w148, element=CameraControlTypeDef."Trigger Mode" ("Enum")) -> ()  [unwired: 2 in, 3 out]
          }
          event "Internal Line Interval": Value Change {
            n118 = event-data() -> ("OldVal"=w158:dbl)  [unwired: 1 in, 5 out]
            n119 = Enqueue Element(queue=w159, element=CameraControlTypeDef."IntervalLineInt", timeout in ms (-1)=w158) -> ()  [unwired: 1 in, 3 out]
          }
        }
      }
      n120 = disable-structure shown="Disabled" {
        disable-tunnel: 0.0 -> [w601 _]
        disable-tunnel: w97 -> [w600 _]
        disable-tunnel: 0 -> [w599 _]
        disable-tunnel: [w598 _] -> _
        disable-tunnel: [w597 _] -> _
        disable-tunnel: w32 -> [w596 _]
        disable-tunnel: w31 -> [w595 _]
        disable-tunnel: w30 -> [w594 _]
        disable-tunnel: w29 -> [w593 _]
        disable-tunnel: w18 -> [w592 _]
        frame Disabled {
          n121 = while {
            tunnel: w593 -> [w615]
            tunnel: [w613] -> w597
            tunnel: [w612] -> w598
            shift-right: [w622] -> _
            shift-left: w600 -> [w620]
            shift-right: [w623] -> _
            shift-left: w601 -> [w621]
            shift-right: [w614] -> _
            shift-left: w600 -> [w618]
            tunnel: w594 -> [w616]
            tunnel: w600 -> [w619]
            shift-right: [w611] -> _
            shift-left: w595 -> [w617]
            shift-right: [w609] -> _
            shift-left: w599 -> [w610]
            tunnel: w592 -> [w608]
            shift-right: [w606] -> _
            shift-left: _ -> [w605]
            tunnel: w596 -> [w604]
            stop <- w624 stop-if-true
            n122 = event shown="[8] \"HardDisk Record\": Value Change" {
              selector: _ -> [_ _ _ _ _ _ _ _ _ _ _ _]
              dyn-events: _ -> [_ _ _ _ _ _ _ _ _ _ _ _]
              timeout: 0 -> [_ _ _ _ _ _ _ _ _ _ _ _]
              tunnel: [w635 w704 w718 w731 w750 w770 w792 w820 w917 w1011 w1047 w1092] -> w623
              tunnel: [w634 w705 w719 w732 w751 w771 w793 w821 w918 w1012 w1048 w1093] -> w622
              tunnel: w621 -> [w646 w704 w718 w731 w750 w770 w792 w820 w917 w1011 w1047 w1092]
              tunnel: w620 -> [w637 w705 w719 w732 w751 w771 w793 w821 w918 w1012 w1048 w1093]
              tunnel: w619 -> [w642 _ _ _ _ _ _ _ _ _ _ _]
              tunnel: w618 -> [w647 w706 w720 w733 w752 w772 w794 w816 w913 w1013 w1055 w1100]
              tunnel: w617 -> [w641 w703 w717 w730 _ w769 _ w817 w914 _ _ _]
              tunnel: w616 -> [w649 w699 w712 w726 w745 w763 w785 w824 w921 w1008 w1024 w1062]
              tunnel: w615 -> [w648 w701 w708 w727 w744 w766 w784 w825 w922 w1007 w1023 w1061]
              tunnel: [w645 w706 w720 w733 w752 w772 w794 w816 w913 w1013 w1055 w1100] -> w614
              tunnel: [w644 w696 w715 w723 w736 w756 w775 w822 w919 w1002 w1050 w1095] -> w613
              tunnel: [w643 w695 w714 w722 w735 w755 w773 w823 w920 w1003 w1051 w1096] -> w612
              tunnel: [w640 w703 w717 w730 w739 w769 w780 w818 w915 w1001 w1049 w1094] -> w611
              tunnel: w610 -> [w632 w702 w716 w729 w749 w768 w791 w819 w916 w1000 w1020 w1056]
              tunnel: [w631 w702 w716 w729 w749 w768 w791 w819 w916 w1000 w1020 w1056] -> w609
              tunnel: w608 -> [w626 _ _ _ _ _ _ w815 w912 _ _ _]
              tunnel: [_ _ _ _ _ _ _ w814 w911 _ _ _] -> w607
              tunnel: w604 -> [w629 _ _ _ _ _ _ w812 _ _ _ _]
              tunnel: [w628 _ _ _ _ _ _ _ _ _ _ _] -> w606
              tunnel: w605 -> [w627 _ _ _ _ _ _ w813 _ _ _ _]
              event Timeout {
                n123 = event-data() -> ()  [unwired: 1 in, 2 out]
                n124 = call <userlib>:"tm_waitnextframe.vi"("error in (no error)"=w648, "Handle in"=w649) -> ("error out"=w652:errorcluster, "Frame Count"=w633:i32, "Frame Index"=w651:i32, "Handle out"=w653:u32)  [unwired: 6 in]
                "Total Frames" <- w633
                n125 = Tick Count (ms)() -> (millisecond timer value=w639:u32)
                n126 = Increment(x=w646) -> (x+1=w636:dbl)
                n127 = Subtract(x=w639, y=w642) -> (x-y=→"Elapsed Time":u32)
                n128 = Add(x=w637, y=u32 1000) -> (x+y=w657:u32)
                n129 = Less Or Equal?(x=w657, y=w639) -> (x <= y?=w638:bool)
                n130 = Add(x=w647, y=u32 50) -> (x+y=w655:u32)
                n131 = Less Or Equal?(x=w655, y=w639) -> (x <= y?=w630:bool)
                n132 = case shown="True" w638 {
                  tunnel: w637 -> [w660 w669]
                  tunnel: [w660 w666] -> w634
                  tunnel: w636 -> [w659 w672]
                  tunnel: w639 -> [_ w666]
                  tunnel: [w659 0.0] -> w635
                  tunnel: w633 -> [_ w661]
                  tunnel: w632 -> [w658 w664]
                  tunnel: [w658 w661] -> w631
                  frame False {
                  }
                  frame True {
                    n133 = Subtract(x=w666, y=w669) -> (x-y=w668:u32)
                    n134 = Subtract(x=w661, y=w664) -> (x-y=w662:i32)
                    n135 = To Double Precision Float(number=w668) -> (double precision float=w674:dbl)
                    n136 = Divide(x=w674, y=1000.0) -> (x/y=w665:dbl)
                    n137 = To Double Precision Float(number=w662) -> (double precision float=w663:dbl)
                    n138 = Divide(x=w663, y=w665) -> (x/y=→"Camera FPS":dbl)
                    n139 = Divide(x=w672, y=w665) -> (x/y=→"Software FPS":dbl)
                  }
                }
                n140 = case shown="True" w630 {
                  tunnel: w647 -> [w679 _]
                  tunnel: w639 -> [_ w692]
                  tunnel: [w679 w692] -> w645
                  tunnel: w653 -> [w678 w691]
                  tunnel: w641 -> [w676 w686]
                  tunnel: w652 -> [w677 w690]
                  tunnel: [w678 w689] -> w644
                  tunnel: [w677 w688] -> w643
                  tunnel: w651 -> [_ w687]
                  tunnel: [w676 w686] -> w640
                  tunnel: w626 -> [_ w685]
                  tunnel: w629 -> [_ w681]
                  tunnel: [w675 w680] -> w628
                  tunnel: w627 -> [w675 _]
                  frame False {
                  }
                  frame True {
                    n141 = call <userlib>:"tm_getframe_a.vi"("error in (no error)"=w690, "Frame Index"=w687, "Buffer Info"=w686, "Handle in"=w691) -> ("error out"=w688:errorcluster, "Data 16"=w680:u16[][], "Handle out"=w689:u32)  [unwired: 3 in, 2 out]
                    n142 = Bundle By Name(cluster=w681, "State"=Stack_Track."Idle", "Stack Number"=0, "Image"=w680) -> (w682:T4)
                    n143 = Enqueue Element(queue=w685, element=w682) -> ()  [unwired: 2 in, 3 out]
                  }
                }
              }
              event "Exposure": Value Change {
                w694 = u32 2049184 items=["SENSOR MODE"=4212128, "CCD MODE"=4212384, "READOUT MODE"=4211872, "ACTIVE VIEW INDEX"=4343136, "BITS PER CHANNEL"=4342976, "IMAGE PIXEL TYPE"=4343296, "BINNING"=4215968, "EXPOSURE TIME"=2049184, "CONTRAST GAIN"=3163312, "CONTRAST OFFSET"=3163328, "LIGHT MODE"=2114720, "SENSITIVITY"=2114992, "PHOTON IMAGING MODE"=2115200, "HIGH DYNAMIC RANGE MODE"=3163360, "WHITE BALANCE"=3163568, "TEMPERATURE"=2115232, "TEMPERATURE TARGET"=2115264, "SENSOR COOLER FAN"=2115296, "LINEBUNDLE HEIGHT"=4212192, "MECHANICAL SHUTTER"=2115488, "BACK FOCUS POSITION"=8422304, "TRIGGER CONNECTOR"=1066432, "TRIGGER SOURCE"=1066144, "OUTPUT TRIGGER SOURCE"=1852576, "TRIGGER GLOBAL EXPOSURE"=2049680, "FIRST TRIGGER BEHAVIOR"=2049696, "CHANNEL SYNC"=1852352, "READOUT DIRECTION"=4211904, "PRE HSYNC COUNT"=1852704] ("Parameter")
                n144 = event-data() -> ("NewVal"=w700:dbl)  [unwired: 1 in, 2 out]
                n145 = call <userlib>:"tm_setparameter_a.vi"("error in (no error)"=w701, "Value in"=w700, "Parameter"=w694, "Handle in"=w699) -> ("error out"=w698:errorcluster, "Handle out"=w697:u32)  [unwired: 6 in]
                n146 = call <userlib>:"tm_getparameter_a.vi"("error in (no error)"=w698, "Parameter"=w694, "Handle in"=w697) -> ("error out"=w695:errorcluster, "Value out"=w693:dbl, "Handle out"=w696:u32)  [unwired: 6 in]
                n147 = local write "EXP"(w693) -> ()
              }
              event "Internal Line Interval": Value Change {
                w707 = u32 4191424 items=["SENSOR MODE"=4212128, "CCD MODE"=4212384, "READOUT MODE"=4211872, "ACTIVE VIEW INDEX"=4343136, "BITS PER CHANNEL"=4342976, "IMAGE PIXEL TYPE"=4343296, "BINNING"=4215968, "EXPOSURE TIME"=2049184, "CONTRAST GAIN"=3163312, "CONTRAST OFFSET"=3163328, "LIGHT MODE"=2114720, "SENSITIVITY"=2114992, "PHOTON IMAGING MODE"=2115200, "HIGH DYNAMIC RANGE MODE"=3163360, "WHITE BALANCE"=3163568, "TEMPERATURE"=2115232, "TEMPERATURE TARGET"=2115264, "SENSOR COOLER FAN"=2115296, "LINEBUNDLE HEIGHT"=4212192, "MECHANICAL SHUTTER"=2115488, "BACK FOCUS POSITION"=8422304, "TRIGGER CONNECTOR"=1066432, "TRIGGER SOURCE"=1066144, "OUTPUT TRIGGER SOURCE"=1852576, "TRIGGER GLOBAL EXPOSURE"=2049680, "FIRST TRIGGER BEHAVIOR"=2049696, "CHANNEL SYNC"=1852352, "READOUT DIRECTION"=4211904, "PRE HSYNC COUNT"=1852704, "INTERNAL LINE SPEED"=4191408, "INTERNAL LINE INVERVAL"=4191424] ("Parameter")
                n148 = event-data() -> ("NewVal"=w711:dbl)  [unwired: 1 in, 2 out]
                n149 = call <userlib>:"tm_setparameter_a.vi"("error in (no error)"=w708, "Value in"=w711, "Parameter"=w707, "Handle in"=w712) -> ("error out"=w709:errorcluster, "Handle out"=w710:u32)  [unwired: 6 in]
                n150 = call <userlib>:"tm_getparameter_a.vi"("error in (no error)"=w709, "Parameter"=w707, "Handle in"=w710) -> ("error out"=w714:errorcluster, "Value out"=w713:dbl, "Handle out"=w715:u32)  [unwired: 6 in]
                n151 = local write "Internal Line Interval"(w713) -> ()
              }
              event "Trigger Source": Value Change {
                w728 = u32 1066144 items=["SENSOR MODE"=4212128, "CCD MODE"=4212384, "READOUT MODE"=4211872, "ACTIVE VIEW INDEX"=4343136, "BITS PER CHANNEL"=4342976, "IMAGE PIXEL TYPE"=4343296, "BINNING"=4215968, "EXPOSURE TIME"=2049184, "CONTRAST GAIN"=3163312, "CONTRAST OFFSET"=3163328, "LIGHT MODE"=2114720, "SENSITIVITY"=2114992, "PHOTON IMAGING MODE"=2115200, "HIGH DYNAMIC RANGE MODE"=3163360, "WHITE BALANCE"=3163568, "TEMPERATURE"=2115232, "TEMPERATURE TARGET"=2115264, "SENSOR COOLER FAN"=2115296, "LINEBUNDLE HEIGHT"=4212192, "MECHANICAL SHUTTER"=2115488, "BACK FOCUS POSITION"=8422304, "TRIGGER CONNECTOR"=1066432, "TRIGGER SOURCE"=1066144, "OUTPUT TRIGGER SOURCE"=1852576, "TRIGGER GLOBAL EXPOSURE"=2049680, "FIRST TRIGGER BEHAVIOR"=2049696, "CHANNEL SYNC"=1852352, "READOUT DIRECTION"=4211904, "PRE HSYNC COUNT"=1852704] ("Parameter")
                n152 = event-data() -> ("NewVal"=w721:sgl)  [unwired: 1 in, 3 out]
                n153 = call <userlib>:"tm_setparameter_a.vi"("error in (no error)"=w727, "Value in"=w721, "Parameter"=w728, "Handle in"=w726) -> ("error out"=w725:errorcluster, "Handle out"=w724:u32)  [unwired: 6 in]
                n154 = call <userlib>:"tm_getparameter_a.vi"("error in (no error)"=w725, "Parameter"=w728, "Handle in"=w724) -> ("error out"=w722:errorcluster, "Handle out"=w723:u32)  [unwired: 6 in, 1 out]
              }
              event "Trigger Mode": Value Change {
                w740 = 1 items=["Snap", "Sequence"] ("Capture mode")
                n155 = event-data() -> ("NewVal"=w734:sgl)  [unwired: 1 in, 4 out]
                n156 = call <userlib>:"tm_stopcapture.vi"("error in (no error)"=w744, "Handle in"=w745) -> ("error out"=w747:errorcluster, "Handle out"=w746:u32)  [unwired: 8 in]
                n157 = call <userlib>:"tm_unpreparecapture.vi"("error in (no error)"=w747, "Handle in"=w746) -> ("error out"=w743:errorcluster, "Handle out"=w742:u32)  [unwired: 8 in]
                n158 = call <userlib>:"tm_setpropertyvalue.vi"("error in (no error)"=w743, "Value in"=w734, "Property ID"=u32 1049104, "Handle in"=w742) -> ("error out"=w738:errorcluster, "Handle out"=w741:u32)  [unwired: 6 in]
                n159 = call <userlib>:"tm_preparecapture.vi"("Capture mode"=w740, "Handle in"=w741) -> ("Buffer Info"=w739:T9, "Handle out"=w737:u32)  [unwired: 6 in, 2 out]
                n160 = call <userlib>:"tm_startcapture_b.vi"("error in (no error)"=w738, "Handle in"=w737) -> ("error out"=w735:errorcluster, "Handle out"=w736:u32)  [unwired: 8 in]
              }
              event "Readout Direction": Value Change {
                w761 = 1 items=["Snap", "Sequence"] ("Capture mode")
                w754 = u32 4211904 items=["SENSOR MODE"=4212128, "CCD MODE"=4212384, "READOUT MODE"=4211872, "ACTIVE VIEW INDEX"=4343136, "BITS PER CHANNEL"=4342976, "IMAGE PIXEL TYPE"=4343296, "BINNING"=4215968, "EXPOSURE TIME"=2049184, "CONTRAST GAIN"=3163312, "CONTRAST OFFSET"=3163328, "LIGHT MODE"=2114720, "SENSITIVITY"=2114992, "PHOTON IMAGING MODE"=2115200, "HIGH DYNAMIC RANGE MODE"=3163360, "WHITE BALANCE"=3163568, "TEMPERATURE"=2115232, "TEMPERATURE TARGET"=2115264, "SENSOR COOLER FAN"=2115296, "LINEBUNDLE HEIGHT"=4212192, "MECHANICAL SHUTTER"=2115488, "BACK FOCUS POSITION"=8422304, "TRIGGER CONNECTOR"=1066432, "TRIGGER SOURCE"=1066144, "OUTPUT TRIGGER SOURCE"=1852576, "TRIGGER GLOBAL EXPOSURE"=2049680, "FIRST TRIGGER BEHAVIOR"=2049696, "CHANNEL SYNC"=1852352, "READOUT DIRECTION"=4211904, "PRE HSYNC COUNT"=1852704] ("Parameter")
                n161 = event-data() -> ("NewVal"=w753:sgl)  [unwired: 1 in, 3 out]
                n162 = call <userlib>:"tm_stopcapture.vi"("error in (no error)"=w766, "Handle in"=w763) -> ("error out"=w767:errorcluster, "Handle out"=w762:u32)  [unwired: 8 in]
                n163 = call <userlib>:"tm_unpreparecapture.vi"("error in (no error)"=w767, "Handle in"=w762) -> ("error out"=w765:errorcluster, "Handle out"=w764:u32)  [unwired: 8 in]
                n164 = call <userlib>:"tm_setparameter_a.vi"("error in (no error)"=w765, "Value in"=w753, "Parameter"=w754, "Handle in"=w764) -> ("error out"=w758:errorcluster, "Handle out"=w757:u32)  [unwired: 6 in]
                n165 = call <userlib>:"tm_preparecapture.vi"("error in (no error)"=w758, "Capture mode"=w761, "Handle in"=w757) -> ("error out"=w759:errorcluster, "Handle out"=w760:u32)  [unwired: 5 in, 2 out]
                n166 = call <userlib>:"tm_startcapture_b.vi"("error in (no error)"=w759, "Handle in"=w760) -> ("error out"=w755:errorcluster, "Handle out"=w756:u32)  [unwired: 8 in]
              }
              event "Camera Readout Mode", "Slit Width / Lines": Value Change {
                w778 = 1 items=["Snap", "Sequence"] ("Capture mode")
                n167 = event-data() -> ()  [unwired: 1 in, 4 out]
                n168 = call <userlib>:"tm_stopcapture.vi"("error in (no error)"=w784, "Handle in"=w785) -> ("error out"=w786:errorcluster, "Handle out"=w782:u32)  [unwired: 8 in]
                n169 = call <userlib>:"tm_unpreparecapture.vi"("error in (no error)"=w786, "Handle in"=w782) -> ("error out"=w777:errorcluster, "Handle out"=w783:u32)  [unwired: 8 in]
                n170 = call <userlib>:"tm_setpropertyvalue.vi"("error in (no error)"=w777, "Value in"="Camera Readout Mode", "Property ID"=u32 4194832, "Handle in"=w783) -> ("error out"=w787:errorcluster, "Handle out"=w788:u32)  [unwired: 6 in]
                n171 = case shown="12" "Camera Readout Mode" {
                  tunnel: w788 -> [w799 w806]
                  tunnel: [w798 w801] -> w781
                  tunnel: w787 -> [w796 w811]
                  tunnel: [w795 w811] -> w779
                  frame 1, Default {
                    n172 = local read "Exposure"() -> (w797:dbl)
                    n173 = call <userlib>:"tm_setpropertyvalue.vi"("error in (no error)"=w796, "Value in"=w797, "Property ID"=u32 2031888, "Handle in"=w799) -> ("error out"=w795:errorcluster, "Handle out"=w798:u32)  [unwired: 6 in]
                  }
                  frame 12 {
                    n174 = local read "Exposure"() -> (w810:dbl)
                    n175 = local read "SVW"() -> (w808:i32)
                    n176 = formula code="slitExpos=frameInter*LW/(LinesToReadout\n+10+LW);\nlineInter = slitExpos / LW;"("frameInter"=w810, "LW"="Slit Width / Lines", "LinesToReadout"=w808) -> ("slitExpos"=w802:dbl, "lineInter"=w805:dbl)
                    n177 = call <userlib>:"tm_setpropertyvalue.vi"("Value in"=w805, "Property ID"=u32 4208720, "Handle in"=w806) -> ("Handle out"=w804:u32)  [unwired: 7 in, 1 out]
                    n178 = call <userlib>:"tm_setpropertyvalue.vi"("Value in"=w802, "Property ID"=u32 2031888, "Handle in"=w804) -> ("Handle out"=w801:u32)  [unwired: 7 in, 1 out]
                  }
                }
                n179 = call <userlib>:"tm_preparecapture.vi"("error in (no error)"=w779, "Capture mode"=w778, "Handle in"=w781) -> ("error out"=w774:errorcluster, "Buffer Info"=w780:T9, "Handle out"=w776:u32)  [unwired: 5 in, 1 out]
                n180 = call <userlib>:"tm_startcapture_b.vi"("error in (no error)"=w774, "Handle in"=w776) -> ("error out"=w773:errorcluster, "Handle out"=w775:u32)  [unwired: 8 in]
              }
              event "Ram Record": Value Change {
                n181 = event-data() -> ()  [unwired: 1 in, 5 out]
                n182 = case shown="True" "Ram Record" {
                  tunnel: w825 -> [w829 w852]
                  tunnel: w824 -> [w828 w849]
                  tunnel: [w829 w835] -> w823
                  tunnel: [w828 w837] -> w822
                  tunnel: [w827 w836] -> w818
                  tunnel: w817 -> [w827 _]
                  tunnel: w815 -> [_ w840]
                  tunnel: [_ w838] -> w814
                  tunnel: w813 -> [_ w834]
                  tunnel: w812 -> [_ w830]
                  frame False {
                  }
                  frame True {
                    w846 = 0 items=["Snap", "Sequence"] ("Capture mode")
                    # "Max 2500"
                    n183 = Flush Queue(queue=w840) -> (queue out=w839:refnum<queue>)  [unwired: 1 in, 2 out]
                    n184 = call <userlib>:"tm_stopcapture.vi"("error in (no error)"=w852, "Handle in"=w849) -> ("error out"=w851:errorcluster, "Handle out"=w850:u32)  [unwired: 8 in]
                    n185 = Bundle By Name(cluster=w830, "State"=Stack_Track."Start Sequence", "Stack Number"=0, "Image"=w834) -> (w831:T4)
                    n186 = call <userlib>:"tm_unpreparecapture.vi"("error in (no error)"=w851, "Handle in"=w850) -> ("error out"=w847:errorcluster, "Handle out"=w848:u32)  [unwired: 8 in]
                    n187 = call <userlib>:"tm_preparecapture.vi"("error in (no error)"=w847, "Frames"="Frames", "Capture mode"=w846, "Handle in"=w848) -> ("error out"=w845:errorcluster, "Buffer Info"=w843:T9, "Handle out"=w844:u32)  [unwired: 4 in, 1 out]
                    n188 = Enqueue Element(queue=w839, element=w831) -> (queue out=w841:refnum<queue>)  [unwired: 2 in, 2 out]
                    n189 = case shown="No Error" w845 {
                      selector: w845 -> [w877 w898]
                      tunnel: w844 -> [w876 w899]
                      tunnel: "Frames" -> [w872 _]
                      tunnel: [w857 w895] -> w837
                      tunnel: w843 -> [w873 _]
                      tunnel: [w856 w897] -> w835
                      tunnel: w841 -> [w871 w893]
                      tunnel: w830 -> [w870 _]
                      tunnel: [w855 w893] -> _
                      tunnel: [FALSE ("value") w907] -> w838
                      tunnel: [w854 w896] -> w836
                      frame No Error {
                        w862 = 1 items=["Snap", "Sequence"] ("Capture mode")
                        # "Frames in RAM"
                        n190 = call <userlib>:"tm_startcapture_b.vi"("error in (no error)"=w877, "Handle in"=w876) -> ("error out"=w874:errorcluster, "Handle out"=w875:u32)  [unwired: 8 in]
                        n191 = for {
                          N: w872 -> [_]
                          tunnel: w875 -> [w892]
                          tunnel: w874 -> [w891]
                          tunnel: w873 -> [w888]
                          tunnel: [w887] -> w868
                          tunnel: [w886] -> w867
                          tunnel: w871 -> [w884]
                          tunnel: Stack_Track."Collecting" ("Enum") -> [w882]
                          tunnel: w870 -> [w880]
                          tunnel: [w879] -> w861
                          i -> [w881]
                          n192 = call <userlib>:"tm_waitnextframe.vi"("error in (no error)"=w891, "Handle in"=w892) -> ("error out"=w889:errorcluster, "Frame Index"=→"Frame Index":i32, "Handle out"=w890:u32)  [unwired: 6 in, 1 out]
                          n193 = call <userlib>:"tm_getframe_a.vi"("error in (no error)"=w889, "Frame Index"=w881, "Buffer Info"=w888, "Handle in"=w890) -> ("error out"=w886:errorcluster, "Data 16"=w878:u16[][], "Handle out"=w887:u32)  [unwired: 3 in, 2 out]
                          n194 = Bundle By Name(cluster=w880, "State"=w882, "Stack Number"=w881, "Image"=w878) -> (w883:T4)
                          n195 = Enqueue Element(queue=w884, element=w883) -> (queue out=w879:refnum<queue>)  [unwired: 2 in, 2 out]
                        }
                        n196 = call <userlib>:"tm_stopcapture.vi"("error in (no error)"=w867, "Handle in"=w868) -> ("error out"=w865:errorcluster, "Handle out"=w866:u32)  [unwired: 8 in]
                        n197 = call <userlib>:"tm_unpreparecapture.vi"("error in (no error)"=w865, "Handle in"=w866) -> ("error out"=w864:errorcluster, "Handle out"=w863:u32)  [unwired: 8 in]
                        n198 = Enqueue Element(queue=w861, element=T4 {"State"=enum."End", "Stack Number"=0, "Image"=[], "Stacks"=0} ("input cluster")) -> (queue out=w855:refnum<queue>)  [unwired: 2 in, 2 out]
                        n199 = call <userlib>:"tm_preparecapture.vi"("error in (no error)"=w864, "Capture mode"=w862, "Handle in"=w863) -> ("error out"=w859:errorcluster, "Buffer Info"=w854:T9, "Handle out"=w858:u32)  [unwired: 5 in, 1 out]
                        n200 = call <userlib>:"tm_startcapture_b.vi"("error in (no error)"=w859, "Handle in"=w858) -> ("error out"=w856:errorcluster, "Handle out"=w857:u32)  [unwired: 8 in]
                      }
                      frame Error {
                        w902 = 1 items=["Snap", "Sequence"] ("Capture mode")
                        # "Prepare camera failure, likely too many frames in stack"
                        n201 = One Button Dialog(message="Too many frames in stack", button name ("OK")="OK") -> (true=w907:bool)
                        n202 = call <userlib>:"tm_stopcapture.vi"("error in (no error)"=w898, "Handle in"=w899) -> ("error out"=w905:errorcluster, "Handle out"=w906:u32)  [unwired: 8 in]
                        n203 = call <userlib>:"tm_unpreparecapture.vi"("error in (no error)"=w905, "Handle in"=w906) -> ("error out"=w904:errorcluster, "Handle out"=w903:u32)  [unwired: 8 in]
                        n204 = Enqueue Element(queue=w893, element=T4 {"State"=enum."Idle", "Stack Number"=0, "Image"=[], "Stacks"=0} ("input cluster")) -> ()  [unwired: 2 in, 3 out]
                        n205 = call <userlib>:"tm_preparecapture.vi"("error in (no error)"=w904, "Capture mode"=w902, "Handle in"=w903) -> ("error out"=w901:errorcluster, "Buffer Info"=w896:T9, "Handle out"=w900:u32)  [unwired: 5 in, 1 out]
                        n206 = call <userlib>:"tm_startcapture_b.vi"("error in (no error)"=w901, "Handle in"=w900) -> ("error out"=w897:errorcluster, "Handle out"=w895:u32)  [unwired: 8 in]
                      }
                    }
                  }
                }
              }
              event "HardDisk Record": Value Change {
                n207 = event-data() -> ()  [unwired: 1 in, 5 out]
                n208 = case shown="True" "HardDisk Record" {
                  tunnel: w922 -> [w925 w941]
                  tunnel: w921 -> [w924 w938]
                  tunnel: [w925 w928] -> w920
                  tunnel: [w924 w930] -> w919
                  tunnel: [w923 w929] -> w915
                  tunnel: w914 -> [w923 _]
                  tunnel: w912 -> [_ w926]
                  tunnel: [_ w931] -> w911
                  frame False {
                  }
                  frame True {
                    w935 = 0 items=["Snap", "Sequence"] ("Capture mode")
                    # "Max 50"
                    n209 = call <userlib>:"tm_stopcapture.vi"("error in (no error)"=w941, "Handle in"=w938) -> ("error out"=w940:errorcluster, "Handle out"=w939:u32)  [unwired: 8 in]
                    n210 = call <userlib>:"tm_unpreparecapture.vi"("error in (no error)"=w940, "Handle in"=w939) -> ("error out"=w936:errorcluster, "Handle out"=w937:u32)  [unwired: 8 in]
                    n211 = call <userlib>:"tm_preparecapture.vi"("error in (no error)"=w936, "Frames"="Frames", "Capture mode"=w935, "Handle in"=w937) -> ("error out"=w934:errorcluster, "Buffer Info"=w932:T9, "Handle out"=w933:u32)  [unwired: 4 in, 1 out]
                    n212 = case shown="No Error" w934 {
                      selector: w934 -> [w966 w979]
                      tunnel: w933 -> [w952 w980]
                      tunnel: [w955 w976] -> w930
                      tunnel: w932 -> [w963 _]
                      tunnel: [w954 w978] -> w928
                      tunnel: [FALSE ("value") w988] -> w931
                      tunnel: [w953 w977] -> w929
                      tunnel: "Frames" -> [w949 _]
                      tunnel: w926 -> [w943 w974]
                      frame No Error {
                        w958 = 1 items=["Snap", "Sequence"] ("Capture mode")
                        n213 = call <userlib>:"tm_startrecorder.vi"("frames"=w949, "File"="Temp", "Handle in"=w952) -> ("Handle out"=w951:u32)  [unwired: 7 in, 1 out]
                        n214 = call <userlib>:"tm_startcapture_b.vi"("error in (no error)"=w966, "Handle in"=w951) -> ("error out"=w964:errorcluster, "Handle out"=w965:u32)  [unwired: 8 in]
                        n215 = while {
                          tunnel: w965 -> [w972]
                          tunnel: w964 -> [w971]
                          tunnel: w963 -> [_]
                          tunnel: [w973] -> w961
                          tunnel: w949 -> [w968]
                          stop <- w969 stop-if-true
                          n216 = Wait (ms)(milliseconds to wait=u32 50) -> ()  [unwired: 1 out]
                          n217 = call <userlib>:"tm_getrecorderstatus.vi"("error in (no error)"=w971, "Handle"=w972) -> ("error out"=w973:errorcluster, "Count"=w967:i32)  [unwired: 6 in, 2 out]
                          n218 = Equal?(x=w967, y=w968) -> (x = y?=w969:bool)
                        }
                        n219 = call <userlib>:"tm_stopcapture.vi"("error in (no error)"=w961) -> ("error out"=w948:errorcluster, "Handle out"=w947:u32)  [unwired: 9 in]
                        n220 = call <userlib>:"tm_stoprecorder.vi"("error in (no error)"=w948, "Handle in"=w947) -> ("error out"=w945:errorcluster, "Handle out"=w946:u32)  [unwired: 8 in]
                        n221 = Enqueue Element(queue=w943, element=T4 {"State"=enum."Read Disk", "Stack Number"=0, "Image"=[], "Stacks"=0}, error in (no error)=w945) -> (error out=w944:errorcluster)  [unwired: 1 in, 2 out]
                        n222 = call <userlib>:"tm_unpreparecapture.vi"("error in (no error)"=w944, "Handle in"=w946) -> ("error out"=w960:errorcluster, "Handle out"=w959:u32)  [unwired: 8 in]
                        n223 = call <userlib>:"tm_preparecapture.vi"("error in (no error)"=w960, "Capture mode"=w958, "Handle in"=w959) -> ("error out"=w957:errorcluster, "Buffer Info"=w953:T9, "Handle out"=w956:u32)  [unwired: 5 in, 1 out]
                        n224 = call <userlib>:"tm_startcapture_b.vi"("error in (no error)"=w957, "Handle in"=w956) -> ("error out"=w954:errorcluster, "Handle out"=w955:u32)  [unwired: 8 in]
                      }
                      frame Error {
                        w983 = 1 items=["Snap", "Sequence"] ("Capture mode")
                        # "Prepare camera failure, likely too many frames in stack"
                        n225 = One Button Dialog(message="Too many frames in stack", button name ("OK")="OK") -> (true=w988:bool)
                        n226 = call <userlib>:"tm_stopcapture.vi"("error in (no error)"=w979, "Handle in"=w980) -> ("error out"=w986:errorcluster, "Handle out"=w987:u32)  [unwired: 8 in]
                        n227 = call <userlib>:"tm_unpreparecapture.vi"("error in (no error)"=w986, "Handle in"=w987) -> ("error out"=w985:errorcluster, "Handle out"=w984:u32)  [unwired: 8 in]
                        n228 = Enqueue Element(queue=w974, element=T4 {"State"=enum."STOP", "Stack Number"=0, "Image"=[], "Stacks"=0} ("input cluster")) -> ()  [unwired: 2 in, 3 out]
                        n229 = call <userlib>:"tm_preparecapture.vi"("error in (no error)"=w985, "Capture mode"=w983, "Handle in"=w984) -> ("error out"=w982:errorcluster, "Buffer Info"=w977:T9, "Handle out"=w981:u32)  [unwired: 5 in, 1 out]
                        n230 = call <userlib>:"tm_startcapture_b.vi"("error in (no error)"=w982, "Handle in"=w981) -> ("error out"=w978:errorcluster, "Handle out"=w976:u32)  [unwired: 8 in]
                      }
                    }
                  }
                }
              }
              event "Scan Mode": Value Change {
                w991 = u32 4211872 items=["SENSOR MODE"=4212128, "CCD MODE"=4212384, "READOUT MODE"=4211872, "ACTIVE VIEW INDEX"=4343136, "BITS PER CHANNEL"=4342976, "IMAGE PIXEL TYPE"=4343296, "BINNING"=4215968, "EXPOSURE TIME"=2049184, "CONTRAST GAIN"=3163312, "CONTRAST OFFSET"=3163328, "LIGHT MODE"=2114720, "SENSITIVITY"=2114992, "PHOTON IMAGING MODE"=2115200, "HIGH DYNAMIC RANGE MODE"=3163360, "WHITE BALANCE"=3163568, "TEMPERATURE"=2115232, "TEMPERATURE TARGET"=2115264, "SENSOR COOLER FAN"=2115296, "LINEBUNDLE HEIGHT"=4212192, "MECHANICAL SHUTTER"=2115488, "BACK FOCUS POSITION"=8422304, "TRIGGER CONNECTOR"=1066432, "TRIGGER SOURCE"=1066144, "OUTPUT TRIGGER SOURCE"=1852576, "TRIGGER GLOBAL EXPOSURE"=2049680, "FIRST TRIGGER BEHAVIOR"=2049696, "CHANNEL SYNC"=1852352, "READOUT DIRECTION"=4211904, "PRE HSYNC COUNT"=1852704] ("Parameter")
                w1006 = 1 items=["Snap", "Sequence"] ("Capture mode")
                n231 = event-data() -> ("NewVal"=w996:dbl)  [unwired: 1 in, 2 out]
                n232 = call <userlib>:"tm_stopcapture.vi"("error in (no error)"=w1007, "Handle in"=w1008) -> ("error out"=w1009:errorcluster, "Handle out"=w1010:u32)  [unwired: 8 in]
                n233 = call <userlib>:"tm_unpreparecapture.vi"("error in (no error)"=w1009, "Handle in"=w1010) -> ("error out"=w994:errorcluster, "Handle out"=w995:u32)  [unwired: 8 in]
                n234 = call <userlib>:"tm_setparameter_a.vi"("error in (no error)"=w994, "Value in"=w996, "Parameter"=w991, "Handle in"=w995) -> ("error out"=w993:errorcluster, "Handle out"=w992:u32)  [unwired: 6 in]
                n235 = call <userlib>:"tm_getparameter_a.vi"("error in (no error)"=w993, "Parameter"=w991, "Handle in"=w992) -> ("error out"=w999:errorcluster, "Value out"=w998:dbl, "Handle out"=w997:u32)  [unwired: 6 in]
                n236 = local write "SMD"(w998) -> ()
                n237 = call <userlib>:"tm_preparecapture.vi"("error in (no error)"=w999, "Capture mode"=w1006, "Handle in"=w997) -> ("error out"=w1004:errorcluster, "Buffer Info"=w1001:T9, "Handle out"=w1005:u32)  [unwired: 5 in, 1 out]
                n238 = call <userlib>:"tm_startcapture_b.vi"("error in (no error)"=w1004, "Handle in"=w1005) -> ("error out"=w1003:errorcluster, "Handle out"=w1002:u32)  [unwired: 8 in]
              }
              event "Binning": Value Change {
                w1015 = u32 4215968 items=["BINNING"=4215968, "BITS PER CHANNEL"=2, "ACTIVE VIEW INDEX"=3, "CCD MODE"=4, "SENSOR MODE"=5, "READOUT MODE"=6, "EXPOSURE TIME"=7, "CONTRAST GAIN"=8, "CONTRAST OFFSET"=9, "LIGHT MODE"=10, "SENSITIVITY"=11, "WHITE BALANCE"=12, "PHOTON IMAGING MODE"=13, "HIGH DYNAMIC RANGE MODE"=14, "TRIGGER SOURCE"=15, "TRIGGER ACTIVE"=16, "TRIGGER MODE"=17, "TRIGGER POLARITY"=18, "TRIGGER GLOBAL EXPOSURE"=19, "FIRST TRIGGER BEHAVIOR"=20, "TRIGGER TIMES"=21, "OUTPUT TRIGGER POLARITY"=22, "OUTPUT TRIGGER DELAY"=23, "OUTPUT TRIGGER PERIOD"=24, "TEMPERATURE"=25, "TEMPERATURE TARGET"=26, "SENSOR COOLER FAN"=27, "MECHANICAL SHUTTER"=28, "BACK FOCUS POSITION"=29, "FRAMEBUNDLE MODE"=30, "FRAMEBUNDLE NUMBER"=31, "LINEBUNDLE HEIGHT"=32, "TRIGGER CONNECTOR"=33, "IMAGE PIXEL TYPE"=34, "OUTPUT TRIGGER KIND"=35, "READOUT DIRECTION"=36, "CHANNEL SYNC"=37] ("Parameter")
                w1054 = 1 items=["Snap", "Sequence"] ("Capture mode")
                n239 = event-data() -> ("NewVal"=w1016:u16)  [unwired: 1 in, 2 out]
                n240 = call <userlib>:"tm_stopcapture.vi"("error in (no error)"=w1023, "Handle in"=w1024) -> ("error out"=w1021:errorcluster, "Handle out"=w1022:u32)  [unwired: 8 in]
                n241 = call <userlib>:"tm_unpreparecapture.vi"("error in (no error)"=w1021, "Handle in"=w1022) -> ("error out"=w1017:errorcluster, "Handle out"=w1014:u32)  [unwired: 8 in]
                n242 = call <userlib>:"tm_setparameter_a.vi"("error in (no error)"=w1017, "Value in"=w1016, "Parameter"=w1015, "Handle in"=w1014) -> ("error out"=w1018:errorcluster, "Handle out"=w1019:u32)  [unwired: 6 in]
                n243 = call <userlib>:"tm_getarea_a.vi"("error in (no error)"=w1018, "Handle in"=w1019) -> ("error out"=w1042:errorcluster, "V Offset"=w1044:T8, "H Offset"=w1043:T8, "Handle out"=w1041:u32, "H Width"=w1045:T8, "V Width"=w1046:T8)  [unwired: 4 in]
                n244 = Unbundle By Name(w1043) -> ("Value"=w1037:i32, "Minimum"=w1040:i32, "Maximum"=w1039:i32, "Increment"=w1038:i32)
                n245 = Unbundle By Name(w1044) -> ("Value"=w1027:i32, "Minimum"=w1036:i32, "Maximum"=w1035:i32, "Increment"=w1034:i32)
                n246 = Unbundle By Name(w1045) -> ("Value"=w1026:i32, "Minimum"=w1033:i32, "Maximum"=w1032:i32, "Increment"=w1031:i32)
                n247 = Unbundle By Name(w1046) -> ("Value"=w1025:i32, "Minimum"=w1030:i32, "Maximum"=w1029:i32, "Increment"=w1028:i32)
                n248 = property on="H Offset" class="DigNum (strict)"("Value"=w1037, "Minimum"=w1040, "Maximum"=w1039, "Increment"=w1038) -> ()  [unwired: 2 in, 2 out]
                n249 = property on="V Offset" class="DigNum (strict)"("Value"=w1027, "Minimum"=w1036, "Maximum"=w1035, "Increment"=w1034) -> ()  [unwired: 2 in, 2 out]
                n250 = property on="H Width" class="DigNum (strict)"("Value"=w1026, "Minimum"=w1033, "Maximum"=w1032, "Increment"=w1031) -> ()  [unwired: 2 in, 2 out]
                n251 = property on="V Width" class="DigNum (strict)"("Value"=w1025, "Minimum"=w1030, "Maximum"=w1029, "Increment"=w1028) -> ()  [unwired: 2 in, 2 out]
                n252 = local write "SHO"(w1037) -> ()
                n253 = local write "SVO"(w1027) -> ()
                n254 = local write "SHW"(w1026) -> ()
                n255 = local write "SVW"(w1025) -> ()
                n256 = call <userlib>:"tm_preparecapture.vi"("error in (no error)"=w1042, "Capture mode"=w1054, "Handle in"=w1041) -> ("error out"=w1052:errorcluster, "Buffer Info"=w1049:T9, "Handle out"=w1053:u32)  [unwired: 5 in, 1 out]
                n257 = call <userlib>:"tm_startcapture_b.vi"("error in (no error)"=w1052, "Handle in"=w1053) -> ("error out"=w1051:errorcluster, "Handle out"=w1050:u32)  [unwired: 8 in]
              }
              event "H Offset", "H Width", "V Offset", "V Width": Value Change {
                w1099 = 1 items=["Snap", "Sequence"] ("Capture mode")
                n258 = event-data() -> ()  [unwired: 1 in, 4 out]
                n259 = call <userlib>:"tm_stopcapture.vi"("error in (no error)"=w1061, "Handle in"=w1062) -> ("error out"=w1059:errorcluster, "Handle out"=w1060:u32)  [unwired: 8 in]
                n260 = local read "H Offset"() -> (w1065:i32)
                n261 = local read "H Width"() -> (w1066:i32)
                n262 = local read "V Offset"() -> (w1067:i32)
                n263 = local read "V Width"() -> (w1064:i32)
                n264 = call <userlib>:"tm_unpreparecapture.vi"("error in (no error)"=w1059, "Handle in"=w1060) -> ("error out"=w1057:errorcluster, "Handle out"=w1058:u32)  [unwired: 8 in]
                n265 = Bundle("H Offset"=w1065, "V Offset"=w1067, "H Width"=w1066, "V Width"=w1064) -> (w1063:T10)  [unwired: 1 in]
                n266 = call <userlib>:"tm_setarea.vi"("error in (no error)"=w1057, "Sub Region"=w1063, "Handle in"=w1058) -> ("error out"=w1068:errorcluster, "Handle out"=w1069:u32)  [unwired: 7 in]
                n267 = call <userlib>:"tm_getarea_a.vi"("error in (no error)"=w1068, "Handle in"=w1069) -> ("error out"=w1087:errorcluster, "V Offset"=w1089:T8, "H Offset"=w1088:T8, "Handle out"=w1086:u32, "H Width"=w1090:T8, "V Width"=w1091:T8)  [unwired: 4 in]
                n268 = Unbundle By Name(w1088) -> ("Value"=w1082:i32, "Minimum"=w1085:i32, "Maximum"=w1084:i32, "Increment"=w1083:i32)
                n269 = Unbundle By Name(w1089) -> ("Value"=w1072:i32, "Minimum"=w1081:i32, "Maximum"=w1080:i32, "Increment"=w1079:i32)
                n270 = Unbundle By Name(w1090) -> ("Value"=w1071:i32, "Minimum"=w1078:i32, "Maximum"=w1077:i32, "Increment"=w1076:i32)
                n271 = Unbundle By Name(w1091) -> ("Value"=w1070:i32, "Minimum"=w1075:i32, "Maximum"=w1074:i32, "Increment"=w1073:i32)
                n272 = property on="H Offset" class="DigNum (strict)"("Value"=w1082, "Minimum"=w1085, "Maximum"=w1084, "Increment"=w1083) -> ()  [unwired: 2 in, 2 out]
                n273 = property on="V Offset" class="DigNum (strict)"("Value"=w1072, "Minimum"=w1081, "Maximum"=w1080, "Increment"=w1079) -> ()  [unwired: 2 in, 2 out]
                n274 = property on="H Width" class="DigNum (strict)"("Value"=w1071, "Minimum"=w1078, "Maximum"=w1077, "Increment"=w1076) -> ()  [unwired: 2 in, 2 out]
                n275 = property on="V Width" class="DigNum (strict)"("Value"=w1070, "Minimum"=w1075, "Maximum"=w1074, "Increment"=w1073) -> ()  [unwired: 2 in, 2 out]
                n276 = local write "SHO"(w1082) -> ()
                n277 = local write "SVO"(w1072) -> ()
                n278 = local write "SHW"(w1071) -> ()
                n279 = local write "SVW"(w1070) -> ()
                n280 = call <userlib>:"tm_preparecapture.vi"("error in (no error)"=w1087, "Capture mode"=w1099, "Handle in"=w1086) -> ("error out"=w1097:errorcluster, "Buffer Info"=w1094:T9, "Handle out"=w1098:u32)  [unwired: 5 in, 1 out]
                n281 = call <userlib>:"tm_startcapture_b.vi"("error in (no error)"=w1097, "Handle in"=w1098) -> ("error out"=w1096:errorcluster, "Handle out"=w1095:u32)  [unwired: 8 in]
              }
            }
            n282 = local read "stop"() -> (w603:bool)
            n283 = Unbundle By Name(w612) -> ("status"=w625:bool)
            n284 = Compound Arithmetic op=OR(w625, w603, w607) -> (w624:bool)
          }
        }
        frame Enabled {
        }
      }
      n285 = while {
        tunnel: w18 -> [w175]
        tunnel: w21 -> [w178]
        tunnel: w32 -> [w174]
        shift-right: [w173] -> _
        shift-left: w31 -> [w176]
        shift-right: [w172] -> w27
        shift-left: w30 -> [w177]
        tunnel: w29 -> [w171]
        tunnel: [w165] -> w26
        shift-right: [w163] -> _
        shift-left: _ -> [w162]
        shift-right: [w161] -> _
        shift-left: CameraControlTypeDef."Preview" ("Enum") -> [w160]
        stop <- w164 stop-if-true
        n286 = Dequeue Element(queue=w178, timeout in ms (-1)=1) -> (element=w167:T3, timed out?=w169:bool)  [unwired: 1 in, 2 out]
        n287 = case shown="True" w169 {
          tunnel: [w179 w180] -> w168
          tunnel: w167 -> [w179 _]
          tunnel: w160 -> [_ w180]
          frame False {
          }
          frame True {
          }
        }
        n288 = case shown="\"Trigger Mode\"" w168 {
          tunnel: w177 -> [w199 w284 w342 w385 w425 w463 w498 w502 w520 w531 w565 w586 w590]
          tunnel: w176 -> [_ _ _ _ _ w470 w492 w503 _ _ _ _ w589]
          tunnel: w175 -> [w201 w285 _ _ _ _ w497 _ _ _ _ _ _]
          tunnel: w174 -> [w202 w268 _ _ _ _ w496 _ _ _ _ _ _]
          tunnel: [w186 w276 w355 w394 w432 w470 w492 w503 w506 w529 w549 w570 w589] -> w173
          tunnel: [w181 w275 w348 w392 w430 w471 w491 w502 w510 w528 w561 w582 w590] -> w172
          tunnel: w171 -> [w200 w283 w380 w420 w440 w462 w489 w501 w523 w530 w555 w576 w591]
          tunnel: [w187 w272 w354 w393 w431 w469 w490 w501 w511 w527 w560 w581 w591] -> w165
          tunnel: [w192 w278 w341 w384 w424 w461 w488 w500 w505 w526 w547 w568 w588] -> w163
          tunnel: w162 -> [w191 w278 w341 w384 w424 w461 _ w500 w505 w526 w547 w568 w588]
          tunnel: [w190 w277 w340 w383 w423 w460 CameraControlTypeDef."Preview" ("Enum") CameraControlTypeDef."Idle" ("Enum") w504 w525 w546 w567 w587] -> w161
          tunnel: w160 -> [w190 w277 w340 w383 w423 w460 _ _ w504 w525 w546 w567 w587]
          frame "Ram Record" {
            w185 = 1 items=["Snap", "Sequence"] ("Capture mode")
            n289 = call <userlib>:"tm_stopcapture.vi"("error in (no error)"=w200, "Handle in"=w199) -> ("error out"=w198:errorcluster, "Handle out"=w197:u32)  [unwired: 8 in]
            n290 = local read "Stacks"() -> (w184:dbl)
            n291 = call <userlib>:"tm_unpreparecapture.vi"("error in (no error)"=w198, "Handle in"=w197) -> ("error out"=w195:errorcluster, "Handle out"=w196:u32)  [unwired: 8 in]
            n292 = Flush Queue(queue=w201) -> (queue out=w194:refnum<queue>)  [unwired: 1 in, 2 out]
            n293 = for {
              N: w184 -> [_]
              tunnel: w202 -> [w223]
              tunnel: w194 -> [w215]
              tunnel: [w210] -> w193
              tunnel: [w209] -> w192
              tunnel: w191 -> [w208]
              shift-right: [w205] -> w182
              shift-left: w196 -> [w222]
              shift-right: [w203] -> w183
              shift-left: w195 -> [w221]
              w220 = 0 items=["Snap", "Sequence"] ("Capture mode")
              # "Max 2500"
              n294 = local read "Stack Frames"() -> (w211:i32)
              n295 = Bundle By Name(cluster=w223, "State"=Stack_Track."Start Sequence", "Stack Number"=0, "Image"=w208) -> (w212:T4)
              n296 = call <userlib>:"tm_preparecapture.vi"("error in (no error)"=w221, "Frames"=w211, "Capture mode"=w220, "Handle in"=w222) -> ("error out"=w219:errorcluster, "Buffer Info"=w217:T9, "Handle out"=w218:u32)  [unwired: 4 in, 1 out]
              n297 = Enqueue Element(queue=w215, element=w212) -> (queue out=w216:refnum<queue>)  [unwired: 2 in, 2 out]
              n298 = case shown="No Error" w219 {
                selector: w219 -> [w241 w258]
                tunnel: w218 -> [w240 w259]
                tunnel: w211 -> [w236 _]
                tunnel: [w225 w259] -> w206
                tunnel: w217 -> [w237 _]
                tunnel: [w224 w258] -> w204
                tunnel: w216 -> [w235 w261]
                tunnel: w223 -> [w234 _]
                tunnel: [w230 w261] -> _
                tunnel: [FALSE ("value") w263] -> _
                tunnel: [FALSE ("Boolean") _] -> w210
                tunnel: [w227 w260] -> w209
                tunnel: w208 -> [_ w260]
                frame No Error {
                  # "Frames in RAM"
                  n299 = call <userlib>:"tm_startcapture_b.vi"("error in (no error)"=w241, "Handle in"=w240) -> ("error out"=w238:errorcluster, "Handle out"=w239:u32)  [unwired: 8 in]
                  n300 = for {
                    N: w236 -> [_]
                    tunnel: w239 -> [w257]
                    tunnel: w238 -> [w256]
                    tunnel: w237 -> [w253]
                    tunnel: [w252] -> w225
                    tunnel: [w251] -> w224
                    tunnel: w235 -> [w250]
                    tunnel: Stack_Track."Collecting" ("Enum") -> [w248]
                    tunnel: w234 -> [w246]
                    tunnel: [w245] -> w232
                    tunnel: [w243] -> w227
                    tunnel: TRUE ("Boolean") -> [w242]
                    i -> [w247]
                    n301 = local write "Record Ready"(w242) -> ()
                    n302 = call <userlib>:"tm_waitnextframe.vi"("error in (no error)"=w256, "Handle in"=w257) -> ("error out"=w254:errorcluster, "Frame Index"=w244:i32, "Handle out"=w255:u32)  [unwired: 6 in, 1 out]
                    n303 = call <userlib>:"tm_getframe_a.vi"("error in (no error)"=w254, "Frame Index"=w247, "Buffer Info"=w253, "Handle in"=w255) -> ("error out"=w251:errorcluster, "Data 16"=w243:u16[][], "Handle out"=w252:u32)  [unwired: 3 in, 2 out]
                    n304 = Bundle By Name(cluster=w246, "State"=w248, "Stack Number"=w247, "Image"=w243) -> (w249:T4)
                    n305 = Enqueue Element(queue=w250, element=w249) -> (queue out=w245:refnum<queue>)  [unwired: 2 in, 2 out]
                    n306 = local write "Stack Frames"(w244) -> ()
                  }
                  n307 = Enqueue Element(queue=w232, element=T4 {"State"=enum."End", "Stack Number"=0, "Image"=[], "Stacks"=0} ("input cluster")) -> (queue out=w230:refnum<queue>)  [unwired: 2 in, 2 out]
                }
                frame Error {
                  # "Prepare camera failure, likely too many frames in stack"
                  n308 = One Button Dialog(message="Too many frames in stack", button name ("OK")="OK") -> (true=w263:bool)
                  n309 = Enqueue Element(queue=w261, element=T4 {"State"=enum."Idle", "Stack Number"=0, "Image"=[], "Stacks"=0} ("input cluster")) -> ()  [unwired: 2 in, 3 out]
                }
              }
              n310 = call <userlib>:"tm_stopcapture.vi"("error in (no error)"=w204, "Handle in"=w206) -> ("error out"=w207:errorcluster)  [unwired: 8 in, 1 out]
              n311 = call <userlib>:"tm_unpreparecapture.vi"("error in (no error)"=w207) -> ("error out"=w203:errorcluster, "Handle out"=w205:u32)  [unwired: 9 in]
            }
            n312 = local write "Record Ready"(w193) -> ()
            n313 = call <userlib>:"tm_preparecapture.vi"("error in (no error)"=w183, "Capture mode"=w185, "Handle in"=w182) -> ("error out"=w188:errorcluster, "Buffer Info"=w186:T9, "Handle out"=w189:u32)  [unwired: 5 in, 1 out]
            n314 = call <userlib>:"tm_startcapture_b.vi"("error in (no error)"=w188, "Handle in"=w189) -> ("error out"=w187:errorcluster, "Handle out"=w181:u32)  [unwired: 8 in]
          }
          frame "HardDisk Record" {
            w271 = 1 items=["Snap", "Sequence"] ("Capture mode")
            n315 = local read "Stacks"() -> (w270:dbl)
            n316 = call <userlib>:"tm_stopcapture.vi"("error in (no error)"=w283, "Handle in"=w284) -> ("error out"=w282:errorcluster, "Handle out"=w281:u32)  [unwired: 8 in]
            n317 = call <userlib>:"tm_unpreparecapture.vi"("error in (no error)"=w282, "Handle in"=w281) -> ("error out"=w279:errorcluster, "Handle out"=w280:u32)  [unwired: 8 in]
            n318 = for {
              N: w270 -> [_]
              tunnel: w285 -> [w307]
              shift-right: [w289] -> w266
              shift-left: w280 -> [w306]
              shift-right: [w290] -> w267
              shift-left: w279 -> [w305]
              tunnel: path "C:/temp" ("Temp 2") -> [w295]
              tunnel: w268 -> [w297]
              i -> [w293]
              w304 = 0 items=["Snap", "Sequence"] ("Capture mode")
              # "Would add for loop here"
              # "Max 50"
              n319 = local read "Stack Frames"() -> (w301:i32)
              n320 = call "4Digit File Incrementer tmp.vi"("Number"=w293, "path"=w295) -> ("appended path"=w294:path)  [unwired: 9 in]
              n321 = call <userlib>:"tm_preparecapture.vi"("error in (no error)"=w305, "Frames"=w301, "Capture mode"=w304, "Handle in"=w306) -> ("error out"=w303:errorcluster, "Buffer Info"=w302:T9, "Handle out"=w292:u32)  [unwired: 4 in, 1 out]
              n322 = Bundle By Name(cluster=w297, "State"=Stack_Track."Read Disk", "Stack Number"=0, "Image"=u16[][] [], "Stacks"=w293) -> (w296:T4)
              n323 = case shown="No Error" w303 {
                selector: w303 -> [w313 w333]
                tunnel: w292 -> [w320 w334]
                tunnel: w302 -> [w322 _]
                tunnel: [FALSE ("value") w337] -> _
                tunnel: w301 -> [w318 _]
                tunnel: w307 -> [w316 w335]
                tunnel: w294 -> [w314 _]
                tunnel: [w312 w333] -> w286
                tunnel: [w311 w334] -> w287
                tunnel: w296 -> [w308 _]
                frame No Error {
                  n324 = call <userlib>:"tm_startrecorder.vi"("error in (no error)"=w313, "frames"=w318, "File"=w314, "Handle in"=w320) -> ("error out"=w315:errorcluster, "Handle out"=w319:u32)  [unwired: 6 in]
                  n325 = call <userlib>:"tm_startcapture_b.vi"("error in (no error)"=w315, "Handle in"=w319) -> ("error out"=w323:errorcluster, "Handle out"=w324:u32)  [unwired: 8 in]
                  n326 = while {
                    tunnel: w324 -> [w331]
                    tunnel: w323 -> [w330]
                    tunnel: w322 -> [_]
                    tunnel: [w332] -> w309
                    tunnel: w318 -> [w327]
                    tunnel: [w325] -> w310
                    stop <- w328 stop-if-true
                    n327 = Wait (ms)(milliseconds to wait=u32 50) -> ()  [unwired: 1 out]
                    n328 = call <userlib>:"tm_getrecorderstatus.vi"("error in (no error)"=w330, "Handle"=w331) -> ("error out"=w332:errorcluster, "Count"=w326:i32, "Handle"=w325:u32)  [unwired: 6 in, 1 out]
                    n329 = Equal?(x=w326, y=w327) -> (x = y?=w328:bool)
                  }
                  n330 = call <userlib>:"tm_stoprecorder.vi"("error in (no error)"=w309, "Handle in"=w310) -> ("error out"=w317:errorcluster, "Handle out"=w311:u32)  [unwired: 8 in]
                  n331 = Enqueue Element(queue=w316, element=w308, error in (no error)=w317) -> (error out=w312:errorcluster)  [unwired: 1 in, 2 out]
                }
                frame Error {
                  # "Prepare camera failure, likely too many frames in stack"
                  n332 = One Button Dialog(message="Too many frames in stack", button name ("OK")="OK") -> (true=w337:bool)
                  n333 = Enqueue Element(queue=w335, element=T4 {"State"=enum."STOP", "Stack Number"=0, "Image"=[], "Stacks"=0} ("input cluster")) -> ()  [unwired: 2 in, 3 out]
                }
              }
              n334 = call <userlib>:"tm_stopcapture.vi"("error in (no error)"=w286, "Handle in"=w287) -> ("error out"=w291:errorcluster, "Handle out"=w288:u32)  [unwired: 8 in]
              n335 = call <userlib>:"tm_unpreparecapture.vi"("error in (no error)"=w291, "Handle in"=w288) -> ("error out"=w290:errorcluster, "Handle out"=w289:u32)  [unwired: 8 in]
            }
            n336 = call <userlib>:"tm_preparecapture.vi"("error in (no error)"=w267, "Capture mode"=w271, "Handle in"=w266) -> ("error out"=w273:errorcluster, "Buffer Info"=w276:T9, "Handle out"=w274:u32)  [unwired: 5 in, 1 out]
            n337 = call <userlib>:"tm_startcapture_b.vi"("error in (no error)"=w273, "Handle in"=w274) -> ("error out"=w272:errorcluster, "Handle out"=w275:u32)  [unwired: 8 in]
          }
          frame "ROI" {
            w358 = 1 items=["Snap", "Sequence"] ("Capture mode")
            n338 = call <userlib>:"tm_stopcapture.vi"("error in (no error)"=w380, "Handle in"=w342) -> ("error out"=w381:errorcluster, "Handle out"=w382:u32)  [unwired: 8 in]
            n339 = call <userlib>:"tm_unpreparecapture.vi"("error in (no error)"=w381, "Handle in"=w382) -> ("error out"=w344:errorcluster, "Handle out"=w345:u32)  [unwired: 8 in]
            n340 = local read "V Width"() -> (w350:i32)
            n341 = local read "V Offset"() -> (w352:i32)
            n342 = local read "H Width"() -> (w351:i32)
            n343 = local read "H Offset"() -> (w353:i32)
            n344 = Bundle("H Offset"=w353, "V Offset"=w352, "H Width"=w351, "V Width"=w350) -> (w349:T10)  [unwired: 1 in]
            n345 = call <userlib>:"tm_setarea.vi"("error in (no error)"=w344, "Sub Region"=w349, "Handle in"=w345) -> ("error out"=w347:errorcluster, "Handle out"=w346:u32)  [unwired: 7 in]
            n346 = call <userlib>:"tm_getarea_a.vi"("error in (no error)"=w347, "Handle in"=w346) -> ("error out"=w359:errorcluster, "V Offset"=w362:T8, "H Offset"=w363:T8, "Handle out"=w343:u32, "H Width"=w361:T8, "V Width"=w360:T8)  [unwired: 4 in]
            n347 = Unbundle By Name(w363) -> ("Value"=w367:i32, "Minimum"=w364:i32, "Maximum"=w365:i32, "Increment"=w366:i32)
            n348 = Unbundle By Name(w362) -> ("Value"=w377:i32, "Minimum"=w368:i32, "Maximum"=w369:i32, "Increment"=w370:i32)
            n349 = Unbundle By Name(w361) -> ("Value"=w378:i32, "Minimum"=w371:i32, "Maximum"=w372:i32, "Increment"=w373:i32)
            n350 = Unbundle By Name(w360) -> ("Value"=w379:i32, "Minimum"=w374:i32, "Maximum"=w375:i32, "Increment"=w376:i32)
            n351 = property on="H Offset" class="DigNum (strict)"("Value"=w367, "Minimum"=w364, "Maximum"=w365, "Increment"=w366) -> ()  [unwired: 2 in, 2 out]
            n352 = property on="V Offset" class="DigNum (strict)"("Value"=w377, "Minimum"=w368, "Maximum"=w369, "Increment"=w370) -> ()  [unwired: 2 in, 2 out]
            n353 = property on="H Width" class="DigNum (strict)"("Value"=w378, "Minimum"=w371, "Maximum"=w372, "Increment"=w373) -> ()  [unwired: 2 in, 2 out]
            n354 = property on="V Width" class="DigNum (strict)"("Value"=w379, "Minimum"=w374, "Maximum"=w375, "Increment"=w376) -> ()  [unwired: 2 in, 2 out]
            n355 = local write "SHO"(w367) -> ()
            n356 = local write "SVO"(w377) -> ()
            n357 = local write "SHW"(w378) -> ()
            n358 = local write "SVW"(w379) -> ()
            n359 = call <userlib>:"tm_preparecapture.vi"("error in (no error)"=w359, "Capture mode"=w358, "Handle in"=w343) -> ("error out"=w357:errorcluster, "Buffer Info"=w355:T9, "Handle out"=w356:u32)  [unwired: 5 in, 1 out]
            n360 = call <userlib>:"tm_startcapture_b.vi"("error in (no error)"=w357, "Handle in"=w356) -> ("error out"=w354:errorcluster, "Handle out"=w348:u32)  [unwired: 8 in]
          }
          frame "Binning" {
            w397 = 1 items=["Snap", "Sequence"] ("Capture mode")
            w387 = u32 4215968 items=["BINNING"=4215968, "BITS PER CHANNEL"=2, "ACTIVE VIEW INDEX"=3, "CCD MODE"=4, "SENSOR MODE"=5, "READOUT MODE"=6, "EXPOSURE TIME"=7, "CONTRAST GAIN"=8, "CONTRAST OFFSET"=9, "LIGHT MODE"=10, "SENSITIVITY"=11, "WHITE BALANCE"=12, "PHOTON IMAGING MODE"=13, "HIGH DYNAMIC RANGE MODE"=14, "TRIGGER SOURCE"=15, "TRIGGER ACTIVE"=16, "TRIGGER MODE"=17, "TRIGGER POLARITY"=18, "TRIGGER GLOBAL EXPOSURE"=19, "FIRST TRIGGER BEHAVIOR"=20, "TRIGGER TIMES"=21, "OUTPUT TRIGGER POLARITY"=22, "OUTPUT TRIGGER DELAY"=23, "OUTPUT TRIGGER PERIOD"=24, "TEMPERATURE"=25, "TEMPERATURE TARGET"=26, "SENSOR COOLER FAN"=27, "MECHANICAL SHUTTER"=28, "BACK FOCUS POSITION"=29, "FRAMEBUNDLE MODE"=30, "FRAMEBUNDLE NUMBER"=31, "LINEBUNDLE HEIGHT"=32, "TRIGGER CONNECTOR"=33, "IMAGE PIXEL TYPE"=34, "OUTPUT TRIGGER KIND"=35, "READOUT DIRECTION"=36, "CHANNEL SYNC"=37] ("Parameter")
            n361 = local read "Binning"() -> (w419:u16)
            n362 = call <userlib>:"tm_stopcapture.vi"("error in (no error)"=w420, "Handle in"=w385) -> ("error out"=w421:errorcluster, "Handle out"=w422:u32)  [unwired: 8 in]
            n363 = call <userlib>:"tm_unpreparecapture.vi"("error in (no error)"=w421, "Handle in"=w422) -> ("error out"=w390:errorcluster, "Handle out"=w391:u32)  [unwired: 8 in]
            n364 = call <userlib>:"tm_setparameter_a.vi"("error in (no error)"=w390, "Value in"=w419, "Parameter"=w387, "Handle in"=w391) -> ("error out"=w388:errorcluster, "Handle out"=w386:u32)  [unwired: 6 in]
            n365 = call <userlib>:"tm_getarea_a.vi"("error in (no error)"=w388, "Handle in"=w386) -> ("error out"=w398:errorcluster, "V Offset"=w401:T8, "H Offset"=w402:T8, "Handle out"=w389:u32, "H Width"=w400:T8, "V Width"=w399:T8)  [unwired: 4 in]
            n366 = Unbundle By Name(w402) -> ("Value"=w406:i32, "Minimum"=w403:i32, "Maximum"=w404:i32, "Increment"=w405:i32)
            n367 = Unbundle By Name(w401) -> ("Value"=w416:i32, "Minimum"=w407:i32, "Maximum"=w408:i32, "Increment"=w409:i32)
            n368 = Unbundle By Name(w400) -> ("Value"=w417:i32, "Minimum"=w410:i32, "Maximum"=w411:i32, "Increment"=w412:i32)
            n369 = Unbundle By Name(w399) -> ("Value"=w418:i32, "Minimum"=w413:i32, "Maximum"=w414:i32, "Increment"=w415:i32)
            n370 = property on="H Offset" class="DigNum (strict)"("Value"=w406, "Minimum"=w403, "Maximum"=w404, "Increment"=w405) -> ()  [unwired: 2 in, 2 out]
            n371 = property on="V Offset" class="DigNum (strict)"("Value"=w416, "Minimum"=w407, "Maximum"=w408, "Increment"=w409) -> ()  [unwired: 2 in, 2 out]
            n372 = property on="H Width" class="DigNum (strict)"("Value"=w417, "Minimum"=w410, "Maximum"=w411, "Increment"=w412) -> ()  [unwired: 2 in, 2 out]
            n373 = property on="V Width" class="DigNum (strict)"("Value"=w418, "Minimum"=w413, "Maximum"=w414, "Increment"=w415) -> ()  [unwired: 2 in, 2 out]
            n374 = local write "SHO"(w406) -> ()
            n375 = local write "SVO"(w416) -> ()
            n376 = local write "SHW"(w417) -> ()
            n377 = local write "SVW"(w418) -> ()
            n378 = call <userlib>:"tm_preparecapture.vi"("error in (no error)"=w398, "Capture mode"=w397, "Handle in"=w389) -> ("error out"=w396:errorcluster, "Buffer Info"=w394:T9, "Handle out"=w395:u32)  [unwired: 5 in, 1 out]
            n379 = call <userlib>:"tm_startcapture_b.vi"("error in (no error)"=w396, "Handle in"=w395) -> ("error out"=w393:errorcluster, "Handle out"=w392:u32)  [unwired: 8 in]
          }
          frame "Readout Mode" {
            w435 = 1 items=["Snap", "Sequence"] ("Capture mode")
            # "Set mode to Light Shheet\nUse 12"
            # "Currently only uses auto calculate. \nAleks would probably use manual. Add option."
            n380 = call <userlib>:"tm_stopcapture.vi"("error in (no error)"=w440, "Handle in"=w425) -> ("error out"=w441:errorcluster, "Handle out"=w442:u32)  [unwired: 8 in]
            n381 = call <userlib>:"tm_unpreparecapture.vi"("error in (no error)"=w441, "Handle in"=w442) -> ("error out"=w426:errorcluster, "Handle out"=w427:u32)  [unwired: 8 in]
            n382 = local read "Camera Readout Mode"() -> (w438:u16)
            n383 = call <userlib>:"tm_setpropertyvalue.vi"("error in (no error)"=w426, "Value in"=w438, "Property ID"=u32 4194832, "Handle in"=w427) -> ("error out"=w436:errorcluster, "Handle out"=w437:u32)  [unwired: 6 in]
            n384 = case shown="12" w438 {
              tunnel: [w446 w451] -> w429
              tunnel: w437 -> [w445 w452]
              tunnel: w436 -> [w444 w451]
              tunnel: [w443 w450] -> w428
              frame 1, Default {
                n385 = local read "Exposure"() -> (w447:dbl)
                n386 = call <userlib>:"tm_setpropertyvalue.vi"("error in (no error)"=w444, "Value in"=w447, "Property ID"=u32 2031888, "Handle in"=w445) -> ("error out"=w446:errorcluster, "Handle out"=w443:u32)  [unwired: 6 in]
              }
              frame 12 {
                # "Aleks uses 10e-6"
                n387 = local read "Slit Width / Lines"() -> (w449:sgl)
                n388 = local read "Exposure"() -> (w459:dbl)
                n389 = local read "SVW"() -> (w458:i32)
                n390 = formula code="slitExpos=frameInter*LW/(LinesToReadout\n+10+LW);\nlineInter = slitExpos / LW;"("frameInter"=w459, "LW"=w449, "LinesToReadout"=w458) -> ("slitExpos"=w453:dbl, "lineInter"=w456:dbl)
                "Internal Line Interval" <- w456
                n391 = call <userlib>:"tm_setpropertyvalue.vi"("Value in"=w456, "Property ID"=u32 4208720, "Handle in"=w452) -> ("Handle out"=w455:u32)  [unwired: 7 in, 1 out]
                n392 = call <userlib>:"tm_setpropertyvalue.vi"("Value in"=w453, "Property ID"=u32 2031888, "Handle in"=w455) -> ("Handle out"=w450:u32)  [unwired: 7 in, 1 out]
              }
            }
            n393 = call <userlib>:"tm_preparecapture.vi"("error in (no error)"=w429, "Capture mode"=w435, "Handle in"=w428) -> ("error out"=w434:errorcluster, "Buffer Info"=w432:T9, "Handle out"=w433:u32)  [unwired: 5 in, 1 out]
            n394 = call <userlib>:"tm_startcapture_b.vi"("error in (no error)"=w434, "Handle in"=w433) -> ("error out"=w431:errorcluster, "Handle out"=w430:u32)  [unwired: 8 in]
          }
          frame "Update" {
            w467 = u32 1066144 items=["SENSOR MODE"=4212128, "CCD MODE"=4212384, "READOUT MODE"=4211872, "ACTIVE VIEW INDEX"=4343136, "BITS PER CHANNEL"=4342976, "IMAGE PIXEL TYPE"=4343296, "BINNING"=4215968, "EXPOSURE TIME"=2049184, "CONTRAST GAIN"=3163312, "CONTRAST OFFSET"=3163328, "LIGHT MODE"=2114720, "SENSITIVITY"=2114992, "PHOTON IMAGING MODE"=2115200, "HIGH DYNAMIC RANGE MODE"=3163360, "WHITE BALANCE"=3163568, "TEMPERATURE"=2115232, "TEMPERATURE TARGET"=2115264, "SENSOR COOLER FAN"=2115296, "LINEBUNDLE HEIGHT"=4212192, "MECHANICAL SHUTTER"=2115488, "BACK FOCUS POSITION"=8422304, "TRIGGER CONNECTOR"=1066432, "TRIGGER SOURCE"=1066144, "OUTPUT TRIGGER SOURCE"=1852576, "TRIGGER GLOBAL EXPOSURE"=2049680, "FIRST TRIGGER BEHAVIOR"=2049696, "CHANNEL SYNC"=1852352, "READOUT DIRECTION"=4211904, "PRE HSYNC COUNT"=1852704] ("Parameter")
            w472 = u32 2049184 items=["SENSOR MODE"=4212128, "CCD MODE"=4212384, "READOUT MODE"=4211872, "ACTIVE VIEW INDEX"=4343136, "BITS PER CHANNEL"=4342976, "IMAGE PIXEL TYPE"=4343296, "BINNING"=4215968, "EXPOSURE TIME"=2049184, "CONTRAST GAIN"=3163312, "CONTRAST OFFSET"=3163328, "LIGHT MODE"=2114720, "SENSITIVITY"=2114992, "PHOTON IMAGING MODE"=2115200, "HIGH DYNAMIC RANGE MODE"=3163360, "WHITE BALANCE"=3163568, "TEMPERATURE"=2115232, "TEMPERATURE TARGET"=2115264, "SENSOR COOLER FAN"=2115296, "LINEBUNDLE HEIGHT"=4212192, "MECHANICAL SHUTTER"=2115488, "BACK FOCUS POSITION"=8422304, "TRIGGER CONNECTOR"=1066432, "TRIGGER SOURCE"=1066144, "OUTPUT TRIGGER SOURCE"=1852576, "TRIGGER GLOBAL EXPOSURE"=2049680, "FIRST TRIGGER BEHAVIOR"=2049696, "CHANNEL SYNC"=1852352, "READOUT DIRECTION"=4211904, "PRE HSYNC COUNT"=1852704] ("Parameter")
            # "Fails"
            # "Error on get"
            n395 = local read "Exposure"() -> (w474:dbl)
            n396 = disable-structure shown="Disabled" {
              disable-tunnel: w463 -> [w479 _]
              disable-tunnel: w462 -> [w478 _]
              frame Disabled {
                w477 = u32 4226016 items=["SENSOR MODE"=4212128, "CCD MODE"=4212384, "READOUT MODE"=4211872, "ACTIVE VIEW INDEX"=4343136, "BITS PER CHANNEL"=4342976, "IMAGE PIXEL TYPE"=4343296, "BINNING"=4215968, "EXPOSURE TIME"=2049184, "CONTRAST GAIN"=3163312, "CONTRAST OFFSET"=3163328, "LIGHT MODE"=2114720, "SENSITIVITY"=2114992, "PHOTON IMAGING MODE"=2115200, "HIGH DYNAMIC RANGE MODE"=3163360, "WHITE BALANCE"=3163568, "TEMPERATURE"=2115232, "TEMPERATURE TARGET"=2115264, "SENSOR COOLER FAN"=2115296, "LINEBUNDLE HEIGHT"=4212192, "MECHANICAL SHUTTER"=2115488, "BACK FOCUS POSITION"=8422304, "TRIGGER CONNECTOR"=1066432, "TRIGGER SOURCE"=1066144, "OUTPUT TRIGGER SOURCE"=1852576, "TRIGGER GLOBAL EXPOSURE"=2049680, "FIRST TRIGGER BEHAVIOR"=2049696, "CHANNEL SYNC"=1852352, "READOUT DIRECTION"=4211904, "PRE HSYNC COUNT"=1852704, "INTERNAL LINE SPEED"=4226000, "INTERNAL LINE INTERVAL"=4226016] ("Parameter")
                n397 = local read "Internal Line Interval"() -> (w481:dbl)
                n398 = call <userlib>:"tm_setparameter_a.vi"("error in (no error)"=w478, "Value in"=w481, "Parameter"=w477, "Handle in"=w479) -> ("error out"=w480:errorcluster, "Handle out"=w483:u32)  [unwired: 6 in]
                n399 = call <userlib>:"tm_getparameter_a.vi"("error in (no error)"=w480, "Parameter"=w477, "Handle in"=w483) -> ("Value out"=w482:dbl)  [unwired: 6 in, 2 out]
                n400 = local write "Internal Line Interval"(w482) -> ()
              }
              frame Enabled {
              }
            }
            n401 = call <userlib>:"tm_setparameter_a.vi"("error in (no error)"=w462, "Value in"=w474, "Parameter"=w472, "Handle in"=w463) -> ("error out"=w476:errorcluster, "Handle out"=w473:u32)  [unwired: 6 in]
            n402 = call <userlib>:"tm_getparameter_a.vi"("error in (no error)"=w476, "Parameter"=w472, "Handle in"=w473) -> ("Value out"=w475:dbl)  [unwired: 6 in, 2 out]
            n403 = local write "EXP"(w475) -> ()
            n404 = local read "Trigger Source"() -> (w465:sgl)
            n405 = call <userlib>:"tm_setparameter_a.vi"("error in (no error)"=w462, "Value in"=w465, "Parameter"=w467, "Handle in"=w463) -> ("error out"=w464:errorcluster, "Handle out"=w468:u32)  [unwired: 6 in]
            n406 = call <userlib>:"tm_getparameter_a.vi"("error in (no error)"=w464, "Parameter"=w467, "Handle in"=w468) -> ("error out"=w469:errorcluster, "Value out"=w466:dbl, "Handle out"=w471:u32)  [unwired: 6 in]
            n407 = local write "Trigger Source"(w466) -> ()
          }
          frame "Preview", Default {
            # "Slows it all down somewhat"
            # "Currently the external trigger setting means that frames are dropped because the system lingers at this point. \nIdeally I should set it so when the system is external and recording it won't run this section.\n\nThis is what HC Image does, it offers no live video when you switch from live to record mode.\n\nRealistically when tirgger set external and this times out once then ignore this step.\nBut it'd have to be reset after a recording.\n\nNeed to think more betterer about how to handle this else frames will just be dropped. Probably best to just have a seperate scan mode\nOr at least just a boolean to turn off this live capture section. Working now maybe"
            n408 = call <userlib>:"tm_waitnextframe.vi"("error in (no error)"=w489, "Timeout"=3000, "Handle in"=w498) -> ("error out"=w485:errorcluster, "Handle out"=w486:u32)  [unwired: 5 in, 2 out]
            n409 = call <userlib>:"tm_getframe_a.vi"("error in (no error)"=w485, "Buffer Info"=w492, "Handle in"=w486) -> ("error out"=w490:errorcluster, "Data 16"=w488:u16[][], "Handle out"=w491:u32)  [unwired: 4 in, 2 out]
            n410 = Bundle By Name(cluster=w496, "State"=Stack_Track."Idle", "Stack Number"=0, "Image"=w488) -> (w493:T4)
            n411 = Enqueue Element(queue=w497, element=w493) -> ()  [unwired: 2 in, 3 out]
          }
          frame "Idle" {
          }
          frame "Scan Mode" {
            w507 = 1 items=["Snap", "Sequence"] ("Capture mode")
            w516 = u32 4211872 items=["SENSOR MODE"=4212128, "CCD MODE"=4212384, "READOUT MODE"=4211872, "ACTIVE VIEW INDEX"=4343136, "BITS PER CHANNEL"=4342976, "IMAGE PIXEL TYPE"=4343296, "BINNING"=4215968, "EXPOSURE TIME"=2049184, "CONTRAST GAIN"=3163312, "CONTRAST OFFSET"=3163328, "LIGHT MODE"=2114720, "SENSITIVITY"=2114992, "PHOTON IMAGING MODE"=2115200, "HIGH DYNAMIC RANGE MODE"=3163360, "WHITE BALANCE"=3163568, "TEMPERATURE"=2115232, "TEMPERATURE TARGET"=2115264, "SENSOR COOLER FAN"=2115296, "LINEBUNDLE HEIGHT"=4212192, "MECHANICAL SHUTTER"=2115488, "BACK FOCUS POSITION"=8422304, "TRIGGER CONNECTOR"=1066432, "TRIGGER SOURCE"=1066144, "OUTPUT TRIGGER SOURCE"=1852576, "TRIGGER GLOBAL EXPOSURE"=2049680, "FIRST TRIGGER BEHAVIOR"=2049696, "CHANNEL SYNC"=1852352, "READOUT DIRECTION"=4211904, "PRE HSYNC COUNT"=1852704] ("Parameter")
            n412 = call <userlib>:"tm_stopcapture.vi"("error in (no error)"=w523, "Handle in"=w520) -> ("error out"=w522:errorcluster, "Handle out"=w521:u32)  [unwired: 8 in]
            n413 = call <userlib>:"tm_unpreparecapture.vi"("error in (no error)"=w522, "Handle in"=w521) -> ("error out"=w518:errorcluster, "Handle out"=w519:u32)  [unwired: 8 in]
            n414 = local read "Scan Mode"() -> (w517:dbl)
            n415 = call <userlib>:"tm_setparameter_a.vi"("error in (no error)"=w518, "Value in"=w517, "Parameter"=w516, "Handle in"=w519) -> ("error out"=w512:errorcluster)  [unwired: 6 in, 1 out]
            n416 = call <userlib>:"tm_getparameter_a.vi"("error in (no error)"=w512, "Parameter"=w516) -> ("error out"=w513:errorcluster, "Value out"=w515:dbl, "Handle out"=w508:u32)  [unwired: 7 in]
            n417 = local write "SMD"(w515) -> ()
            n418 = call <userlib>:"tm_preparecapture.vi"("error in (no error)"=w513, "Capture mode"=w507, "Handle in"=w508) -> ("error out"=w514:errorcluster, "Buffer Info"=w506:T9, "Handle out"=w509:u32)  [unwired: 5 in, 1 out]
            n419 = call <userlib>:"tm_startcapture_b.vi"("error in (no error)"=w514, "Handle in"=w509) -> ("error out"=w511:errorcluster, "Handle out"=w510:u32)  [unwired: 8 in]
          }
          frame "Trigger Mode" {
            w524 = 1 items=["Snap", "Sequence"] ("Capture mode")
            w532 = u32 1049104 ("Property ID")
            n420 = local read "Trigger Mode"() -> (w537:sgl)
            n421 = call <userlib>:"tm_stopcapture.vi"("error in (no error)"=w530, "Handle in"=w531) -> ("error out"=w536:errorcluster, "Handle out"=w544:u32)  [unwired: 8 in]
            n422 = call <userlib>:"tm_unpreparecapture.vi"("error in (no error)"=w536, "Handle in"=w544) -> ("error out"=w534:errorcluster, "Handle out"=w540:u32)  [unwired: 8 in]
            n423 = call <userlib>:"tm_setpropertyvalue.vi"("error in (no error)"=w534, "Value in"=w537, "Property ID"=w532, "Handle in"=w540) -> ("error out"=w533:errorcluster, "Handle out"=w539:u32)  [unwired: 6 in]
            n424 = call <userlib>:"tm_getpropertyvalue.vi"("error in (no error)"=w533, "Property ID"=w532, "Handle in"=w539) -> ("error out"=w541:errorcluster, "Value in"=w538:sgl, "Handle out"=w542:u32)  [unwired: 6 in]
            n425 = local write "Trigger Mode"(w538) -> ()
            n426 = call <userlib>:"tm_preparecapture.vi"("error in (no error)"=w541, "Capture mode"=w524, "Handle in"=w542) -> ("error out"=w535:errorcluster, "Buffer Info"=w529:T9, "Handle out"=w543:u32)  [unwired: 5 in, 1 out]
            n427 = call <userlib>:"tm_startcapture_b.vi"("error in (no error)"=w535, "Handle in"=w543) -> ("error out"=w527:errorcluster, "Handle out"=w528:u32)  [unwired: 8 in]
          }
          frame "Readout Direction" {
            w545 = u32 4211904 items=["SENSOR MODE"=4212128, "CCD MODE"=4212384, "READOUT MODE"=4211872, "ACTIVE VIEW INDEX"=4343136, "BITS PER CHANNEL"=4342976, "IMAGE PIXEL TYPE"=4343296, "BINNING"=4215968, "EXPOSURE TIME"=2049184, "CONTRAST GAIN"=3163312, "CONTRAST OFFSET"=3163328, "LIGHT MODE"=2114720, "SENSITIVITY"=2114992, "PHOTON IMAGING MODE"=2115200, "HIGH DYNAMIC RANGE MODE"=3163360, "WHITE BALANCE"=3163568, "TEMPERATURE"=2115232, "TEMPERATURE TARGET"=2115264, "SENSOR COOLER FAN"=2115296, "LINEBUNDLE HEIGHT"=4212192, "MECHANICAL SHUTTER"=2115488, "BACK FOCUS POSITION"=8422304, "TRIGGER CONNECTOR"=1066432, "TRIGGER SOURCE"=1066144, "OUTPUT TRIGGER SOURCE"=1852576, "TRIGGER GLOBAL EXPOSURE"=2049680, "FIRST TRIGGER BEHAVIOR"=2049696, "CHANNEL SYNC"=1852352, "READOUT DIRECTION"=4211904, "PRE HSYNC COUNT"=1852704, "INTERNAL LINE SPEED"=4226000, "INTERNAL LINE INTERVAL"=4226016] ("Parameter")
            w556 = 1 items=["Snap", "Sequence"] ("Capture mode")
            n428 = call <userlib>:"tm_stopcapture.vi"("error in (no error)"=w555, "Handle in"=w565) -> ("error out"=w557:errorcluster, "Handle out"=w564:u32)  [unwired: 8 in]
            n429 = call <userlib>:"tm_unpreparecapture.vi"("error in (no error)"=w557, "Handle in"=w564) -> ("error out"=w558:errorcluster, "Handle out"=w563:u32)  [unwired: 8 in]
            n430 = local read "Readout Direction"() -> (w548:sgl)
            n431 = call <userlib>:"tm_setparameter_a.vi"("error in (no error)"=w558, "Value in"=w548, "Parameter"=w545, "Handle in"=w563) -> ("error out"=w552:errorcluster, "Handle out"=w554:u32)  [unwired: 6 in]
            n432 = call <userlib>:"tm_getparameter_a.vi"("error in (no error)"=w552, "Parameter"=w545, "Handle in"=w554) -> ("error out"=w551:errorcluster, "Value out"=w550:dbl, "Handle out"=w553:u32)  [unwired: 6 in]
            n433 = local write "Readout Direction"(w550) -> ()
            n434 = call <userlib>:"tm_preparecapture.vi"("error in (no error)"=w551, "Capture mode"=w556, "Handle in"=w553) -> ("error out"=w559:errorcluster, "Buffer Info"=w549:T9, "Handle out"=w562:u32)  [unwired: 5 in, 1 out]
            n435 = call <userlib>:"tm_startcapture_b.vi"("error in (no error)"=w559, "Handle in"=w562) -> ("error out"=w560:errorcluster, "Handle out"=w561:u32)  [unwired: 8 in]
          }
          frame "IntervalLineInt" {
            w566 = 4226016
            w577 = 1 items=["Snap", "Sequence"] ("Capture mode")
            n436 = call <userlib>:"tm_stopcapture.vi"("error in (no error)"=w576, "Handle in"=w586) -> ("error out"=w578:errorcluster, "Handle out"=w585:u32)  [unwired: 8 in]
            n437 = call <userlib>:"tm_unpreparecapture.vi"("error in (no error)"=w578, "Handle in"=w585) -> ("error out"=w579:errorcluster, "Handle out"=w584:u32)  [unwired: 8 in]
            n438 = local read "Internal Line Interval"() -> (w569:dbl)
            n439 = call <userlib>:"tm_setparameter_a.vi"("error in (no error)"=w579, "Value in"=w569, "Parameter"=w566, "Handle in"=w584) -> ("error out"=w573:errorcluster, "Handle out"=w575:u32)  [unwired: 6 in]
            n440 = call <userlib>:"tm_getparameter_a.vi"("error in (no error)"=w573, "Parameter"=w566, "Handle in"=w575) -> ("error out"=w572:errorcluster, "Value out"=w571:dbl, "Handle out"=w574:u32)  [unwired: 6 in]
            n441 = local write "Internal Line Interval"(w571) -> ()
            n442 = call <userlib>:"tm_preparecapture.vi"("error in (no error)"=w572, "Capture mode"=w577, "Handle in"=w574) -> ("error out"=w580:errorcluster, "Buffer Info"=w570:T9, "Handle out"=w583:u32)  [unwired: 5 in, 1 out]
            n443 = call <userlib>:"tm_startcapture_b.vi"("error in (no error)"=w580, "Handle in"=w583) -> ("error out"=w581:errorcluster, "Handle out"=w582:u32)  [unwired: 8 in]
          }
          frame "Disengage Update" {
          }
        }
        n444 = local read "stop"() -> (w166:bool)
        n445 = Compound Arithmetic op=OR(w166, w165) -> (w164:bool)
      }
      n446 = call <userlib>:"tm_stopcapture.vi"("error in (no error)"=w26, "Handle in"=w27) -> ("error out"=w73:errorcluster, "Handle out"=w74:u32)  [unwired: 8 in]
      n447 = call <userlib>:"tm_unpreparecapture.vi"("error in (no error)"=w73, "Handle in"=w74) -> ("error out"=w72:errorcluster, "Handle out"=w75:u32)  [unwired: 8 in]
      n448 = call <userlib>:"tm_closecamera.vi"("error in (no error)"=w72, "Handle in"=w75) -> ("error out"=w100:errorcluster)  [unwired: 9 in]
      n449 = call <userlib>:"tm_deinitialize.vi"("error in (no error)"=w100) -> ("error out"=w22:errorcluster)  [unwired: 10 in]
      n450 = Release Queue(queue=w21, error in (no error)=w22) -> (error out=w20:errorcluster)  [unwired: 1 in, 2 out]
      n451 = Release Queue(queue=w18, error in (no error)=w20) -> (error out=w19:errorcluster)  [unwired: 1 in, 2 out]
    }
  }
  "error out" <- w3
